vi "Live Capture Functional Stack.5.64bit.vi"() -> ()   [LabVIEW 2014]
uses:
  subvis/Stack Track.ctl
  subvis/Stack_State.ctl
  CameraControlTypeDef.ctl
  Desktop/camtiff/ctiff.llb/__CTIFFNewFileAndStyleUINT16.vi
  Desktop/camtiff/ctiff.llb/__CTIFFAddNewPageUINT16.vi
panel:
  in  "Slit Width / Lines 2":sgl=150.0
  out "Frame Index":i32
  in  "Temp":path=path "C:/temp.tmp"
  in  "Frames":i32=100
  in  "HardDisk Record":bool
  in  "Internal Line Interval":dbl
  in  "Slit Width / Lines":sgl=150.0
  in  "Camera Readout Mode":u16(ring)=12 items=["Full Frame"=1, "Slit Scanning"=12]
  in  "Readout Direction":sgl(ring)=1.0 items=["Forward"=1, "Backward"=2]
  in  "Trigger Mode":sgl(ring)=1.0 items=["Normal"=1, "Start "=6]
  in  "Trigger Source":sgl(ring)=2.0 items=["Internal"=1, "External"=2]
  out "State":T1=enum."Start Sequence"
  out "Image":u16[][](graph)
  out "Saving":bool
  in  "AutoIncrement":bool=TRUE
  in  "Path":path=path "C:/Users/spim/Desktop/Craig Cap/temp/a.tiff"
  in  "Frames":i32=100
  out "Frame Index":i32
  out "error out":errorcluster
  in  "stop":bool
  in  "Ram Record":bool
  out "Total Frames":i32
  out "Elapsed Time":u32
  out "Software FPS":dbl
  out "Camera FPS":dbl
  in  "H Offset":i32 min=0 max=0 step=4
  in  "H Width":i32 min=0 max=2048 step=4
  out "SMD":dbl
  out "SHO":i32
  in  "V Offset":i32 min=0 max=0 step=4
  in  "V Width":i32 min=0 max=2048 step=4
  in  "Binning":u16(ring) items=["1x1"=1, "2x2"=2, "4x4"=4]
  out "SHW":i32
  out "SVO":i32
  out "SVW":i32
  in  "Scan Mode":dbl min=0.0 max=2.0 step=1.0
  in  "Exposure":dbl min=0.0 max=10.000004210526315 step=1e-08
  out "EXP":dbl
  out "Camera Model":string
  out "Camera Version":string
  out "Camera Serial":string
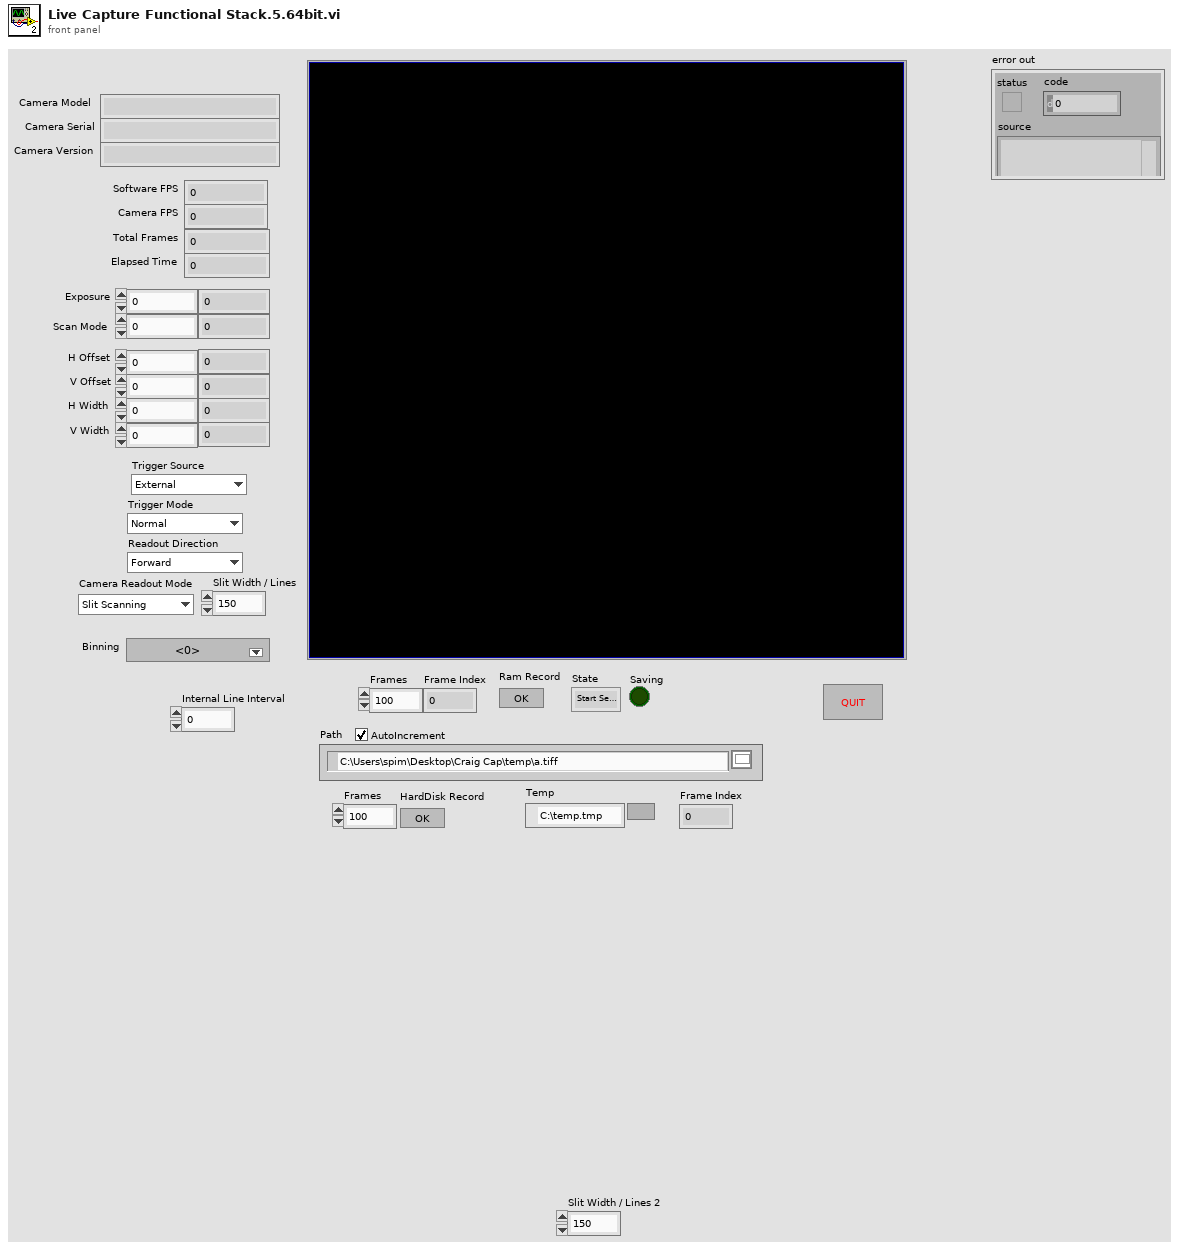
[diagram p1: front panel]
types:
  T1 = typedef "Stack Track.ctl" = enum16{"Idle", "Start Sequence", "Read Disk", "STOP", "Collecting", "End"}
  T2 = typedef "CameraControlTypeDef.ctl" = enum16{"Ram Record", "HardDisk Record", "Disengage Update", "Update", "Idle", "ROI", "Binning", "Scan Mode", "Trigger Mode", "Readout Mode", "Readout Direction"}
  T3 = typedef "Stack_State.ctl" = cluster{"State":T1, "Stack Number":i32, "Image":u16[][]}
  T4 = enum8{"Enabled", "Disabled", "Disabled and Grayed Out"}
  T5 = cluster{"Model":string, "Camera ID":string, "Firmware":string}
  T6 = cluster{"Value":i32, "Minimum":i32, "Maximum":i32, "Increment":i32}
  T7 = cluster{"height":u32, "width":u32, "datatype":u32}
  T8 = cluster{"H Offset":i32, "V Offset":i32, "H Width":i32, "V Width":i32}
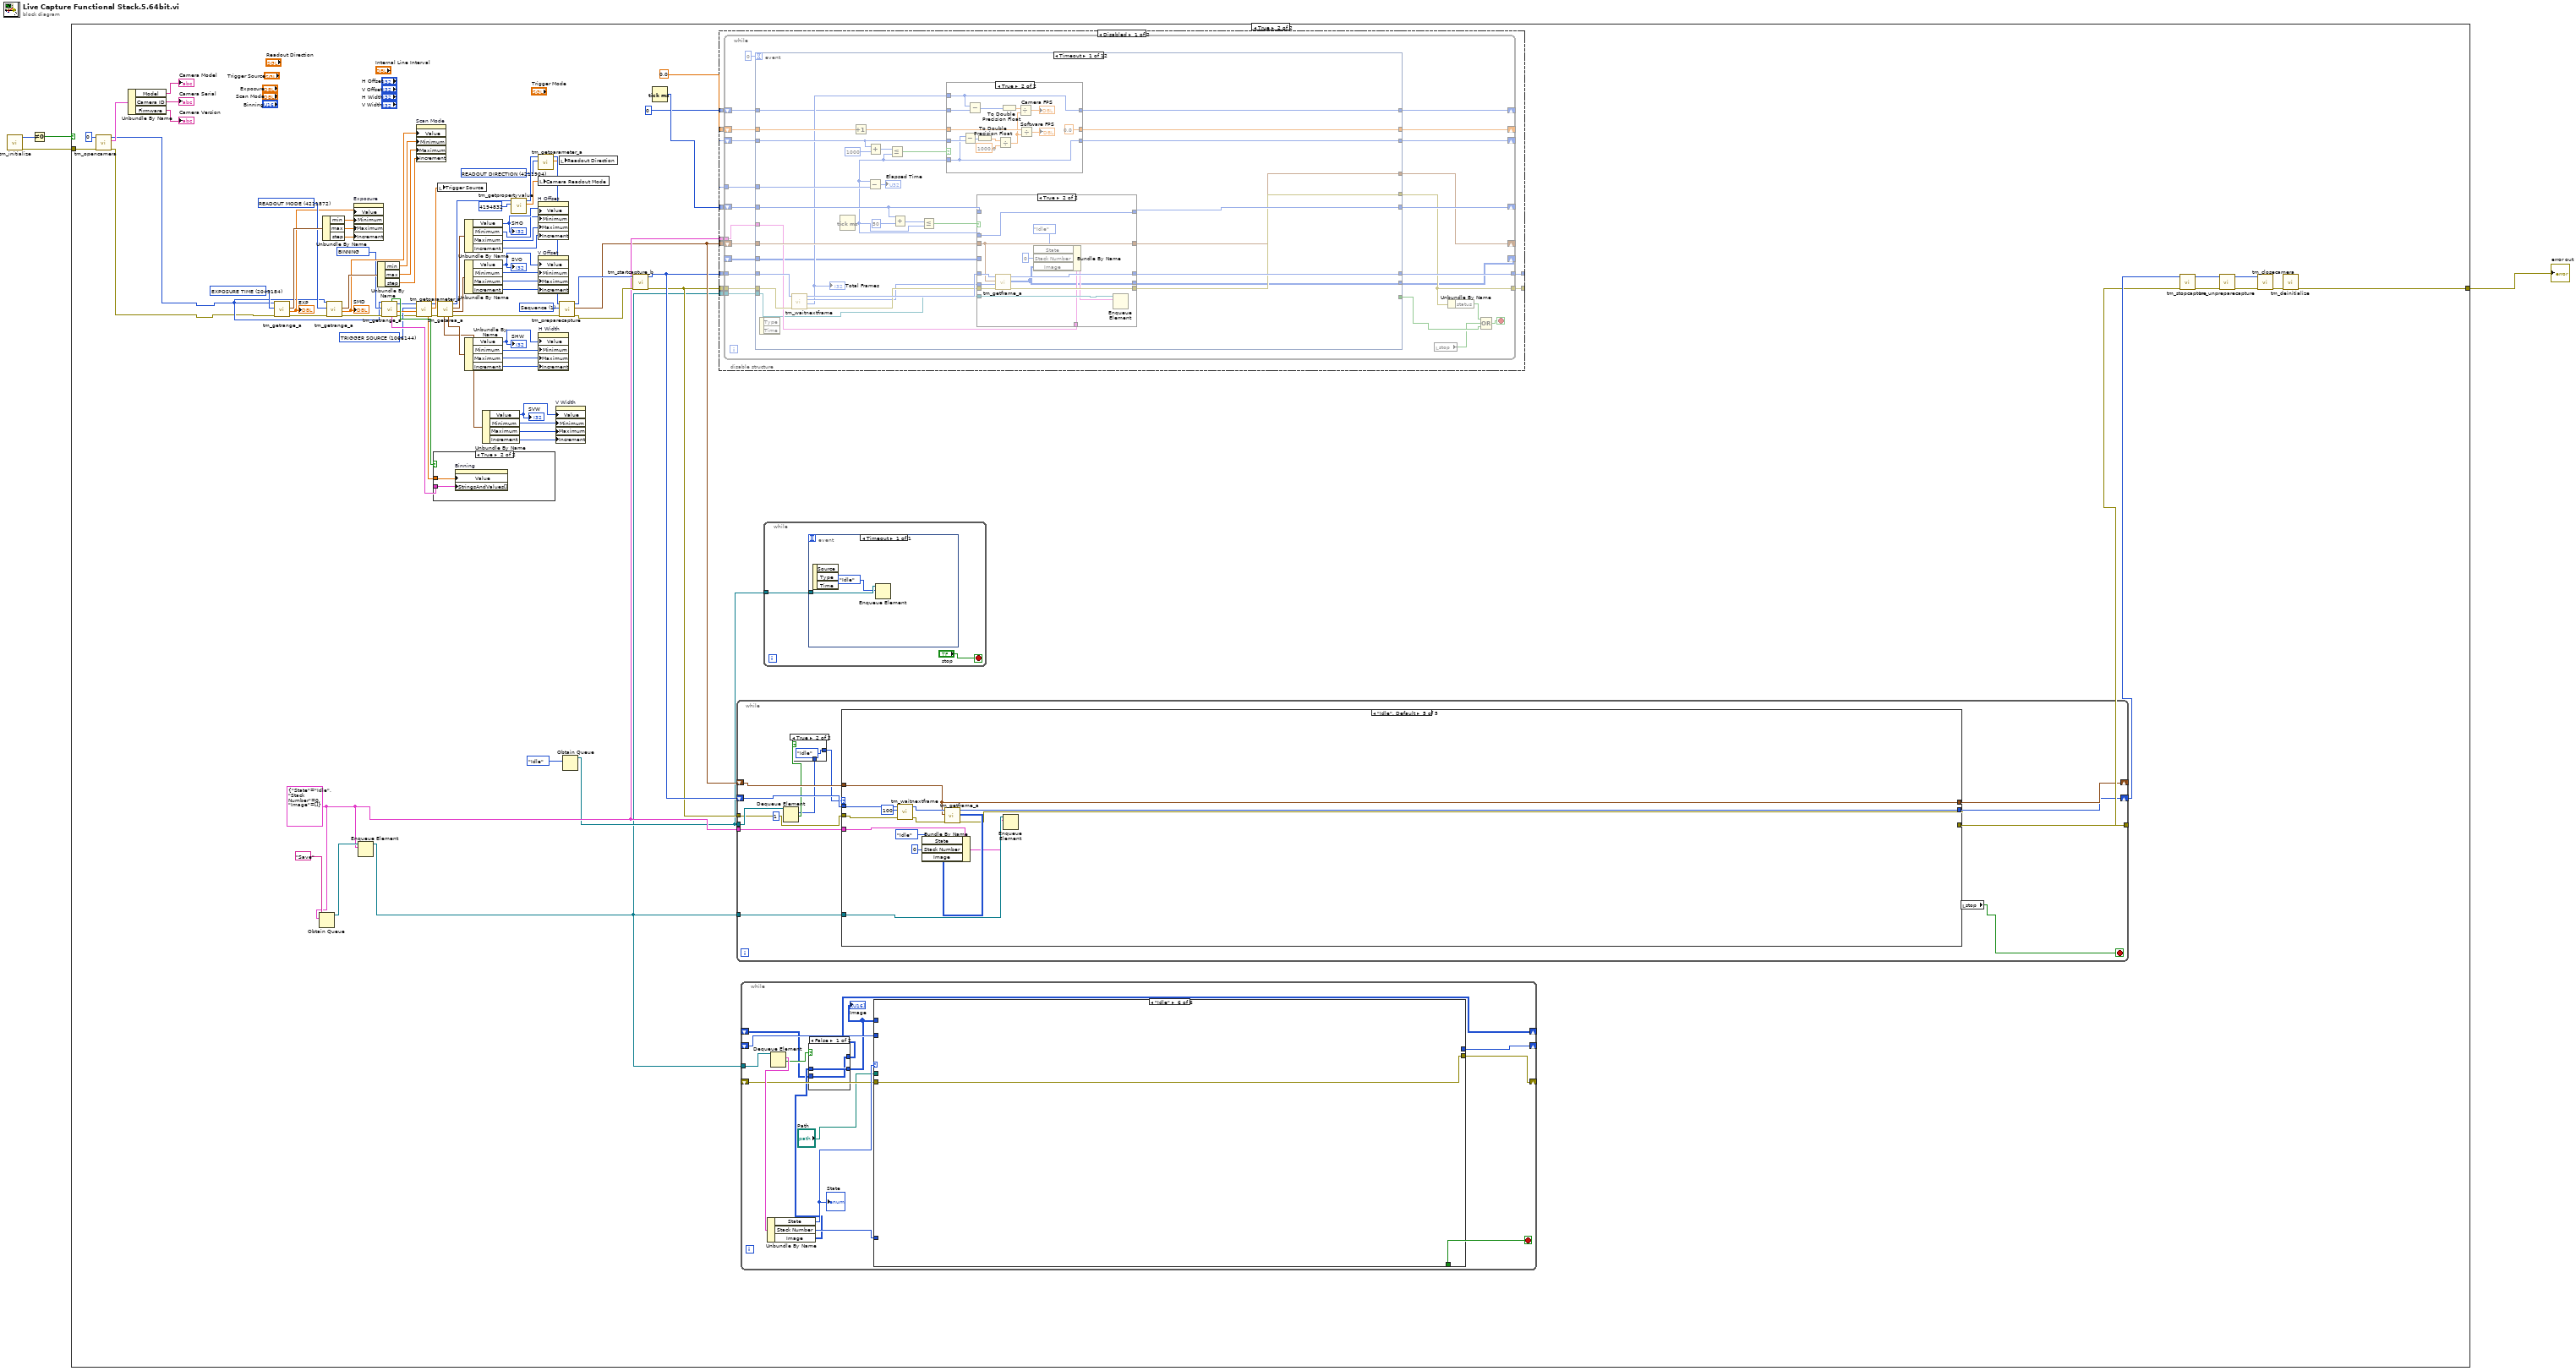
[diagram p0: block diagram]
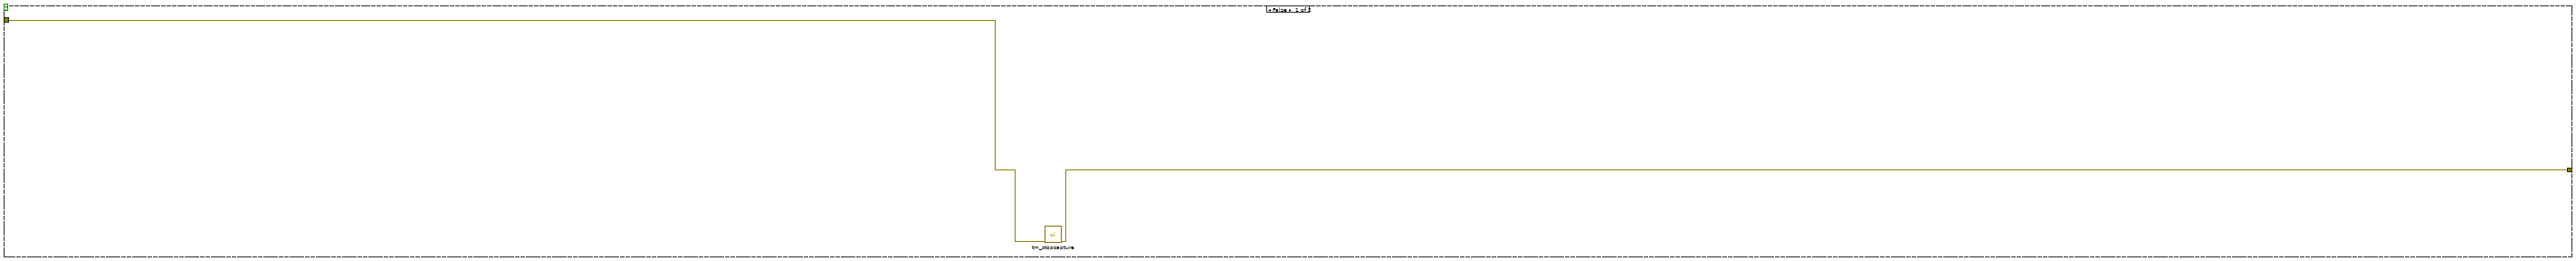
[diagram p2: hidden frame]
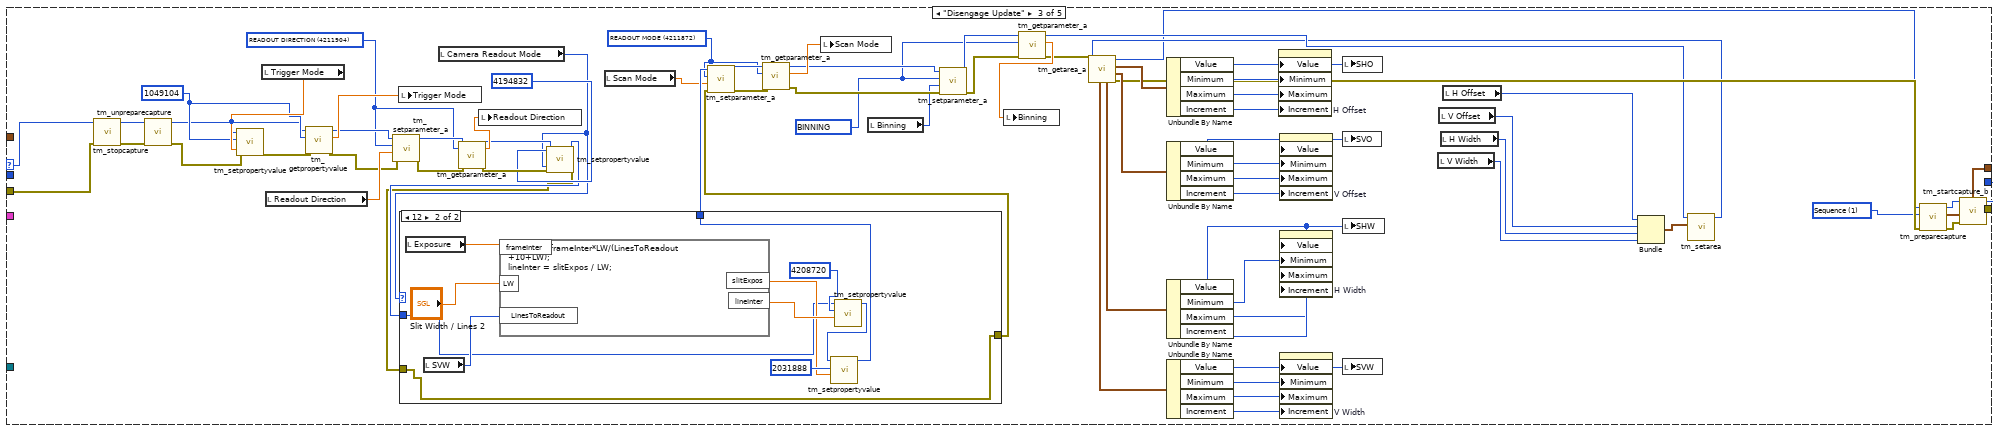
[diagram p6: hidden frame]
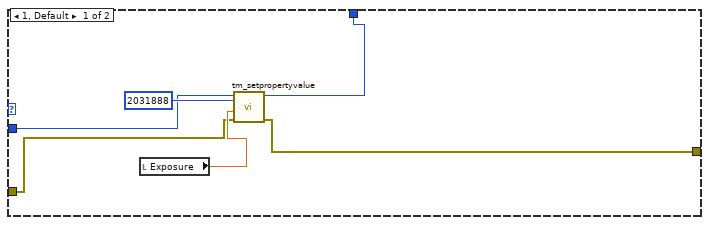
[diagram p7: hidden frame]
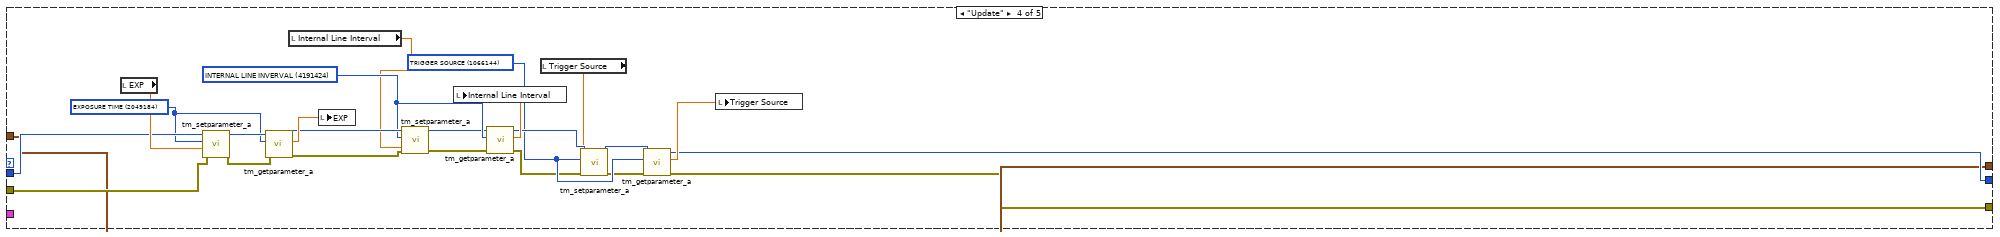
[diagram p8: hidden frame]
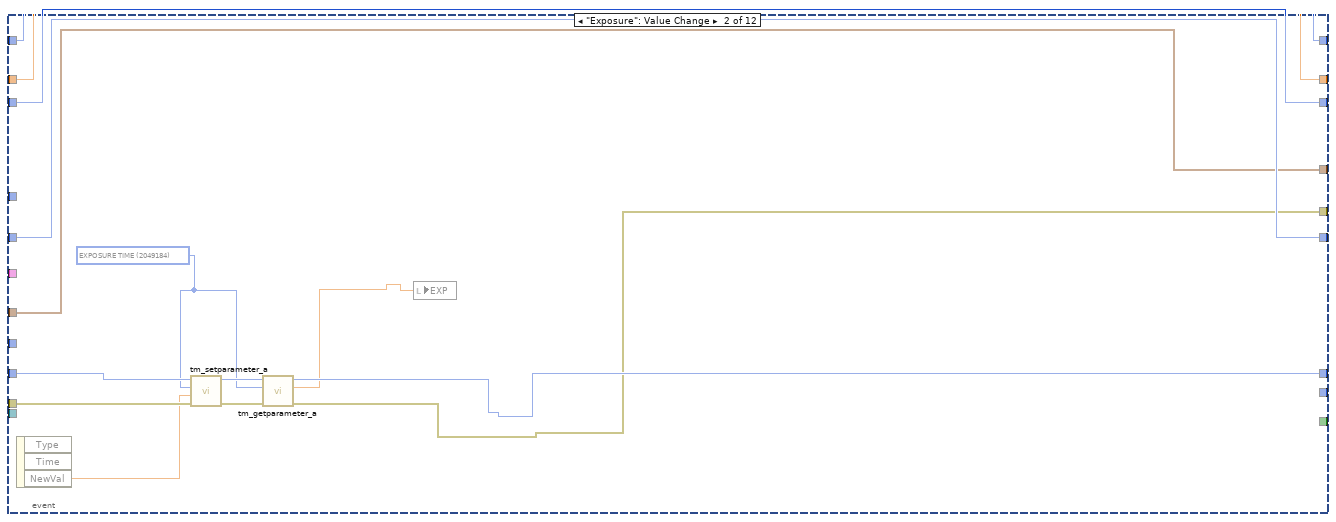
[diagram p11: hidden frame]
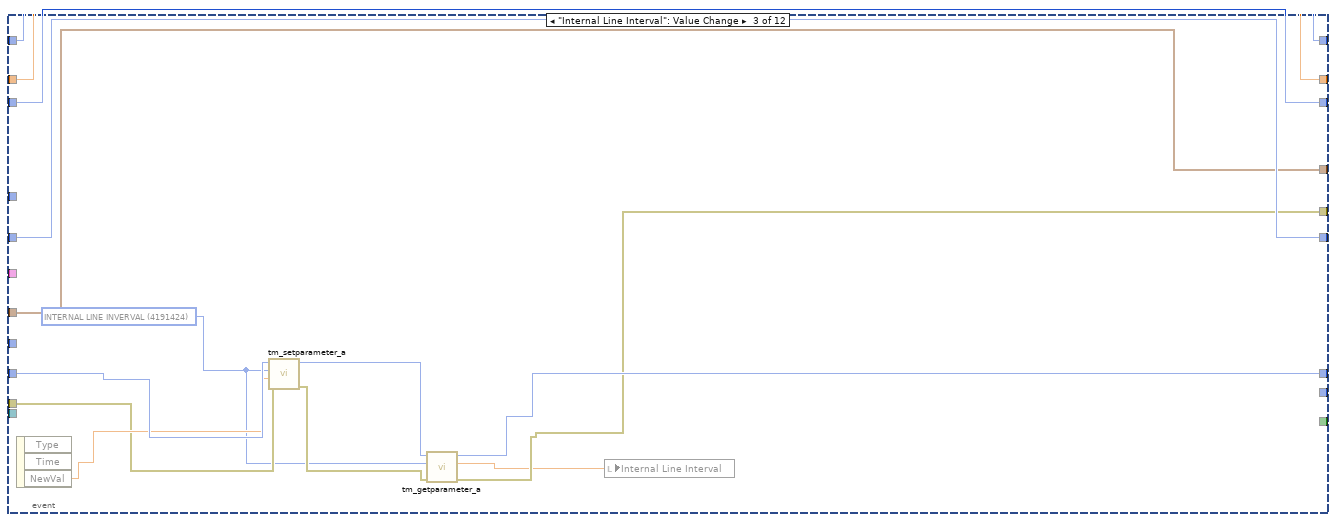
[diagram p12: hidden frame]
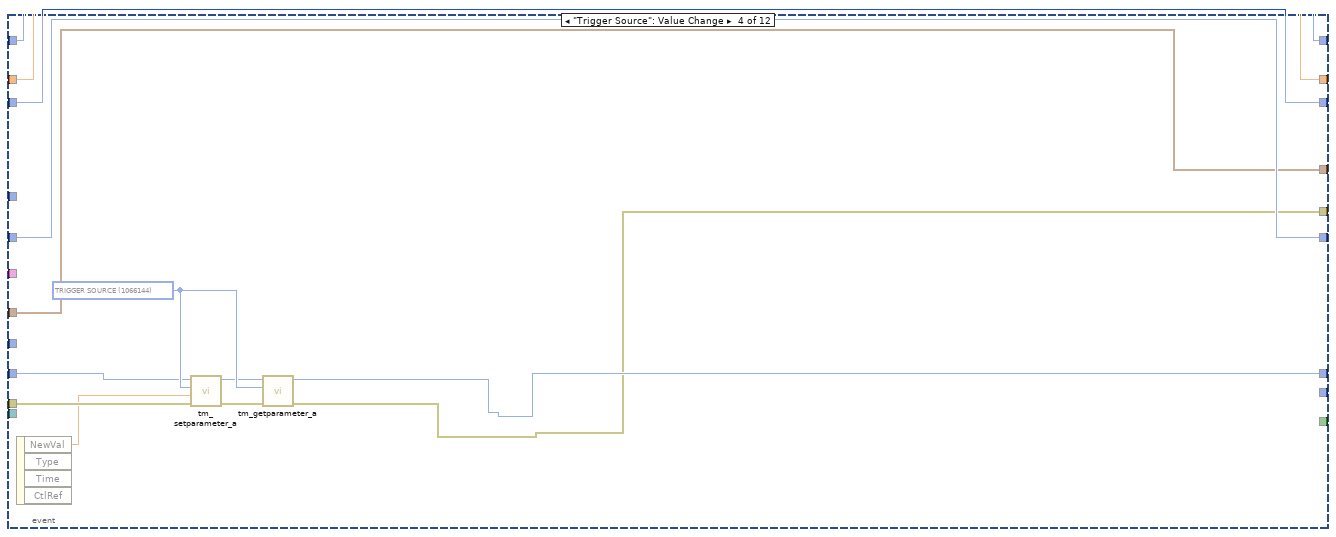
[diagram p13: hidden frame]
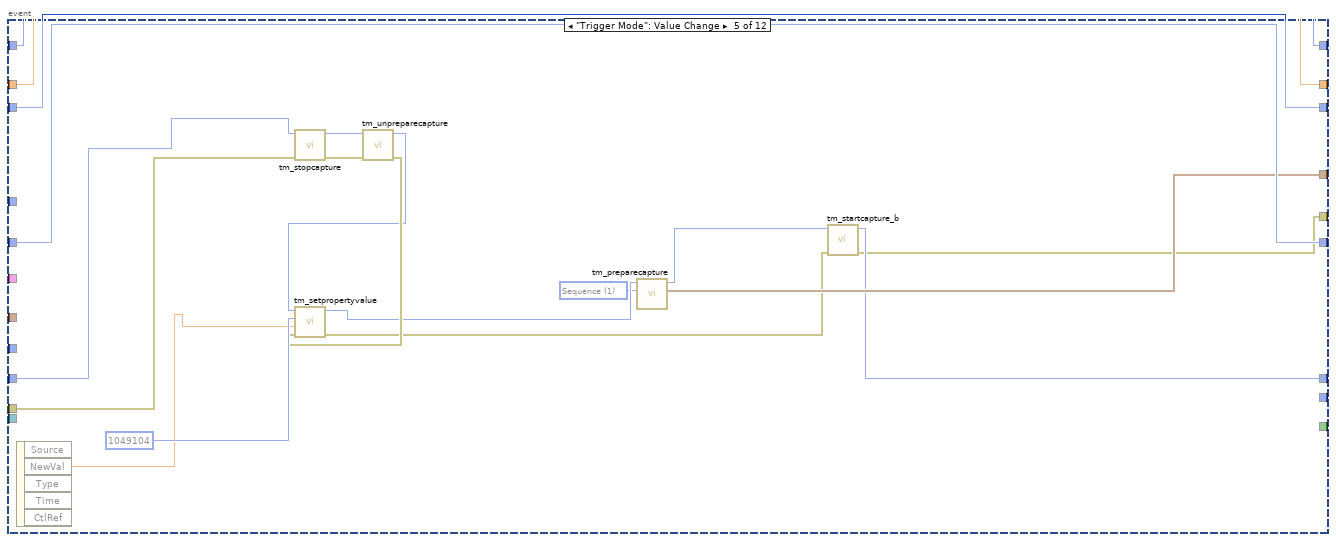
[diagram p14: hidden frame]
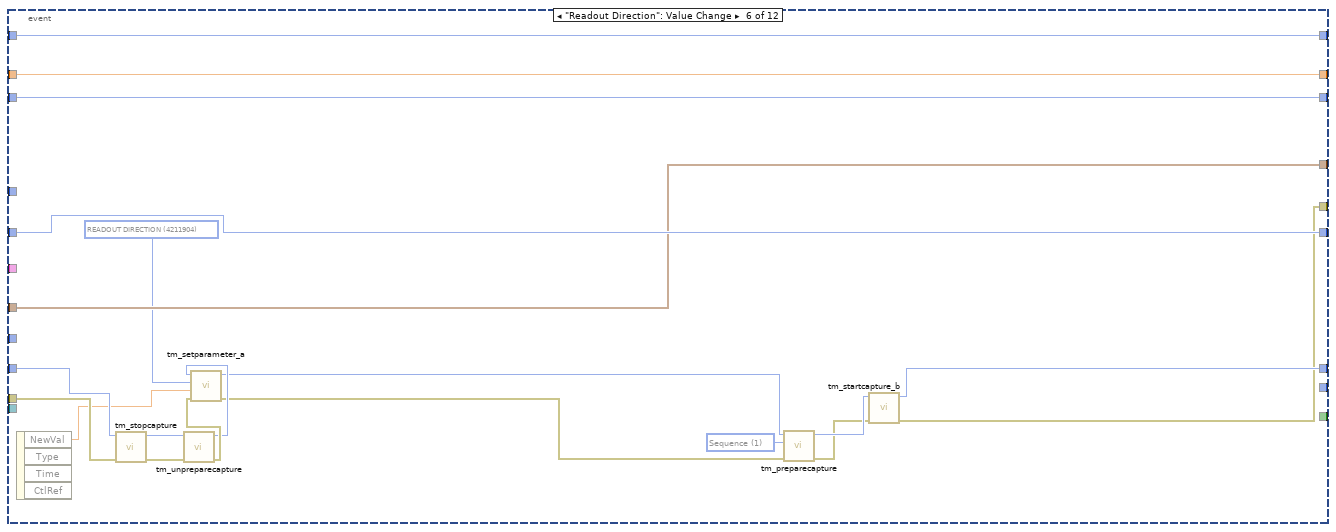
[diagram p15: hidden frame]
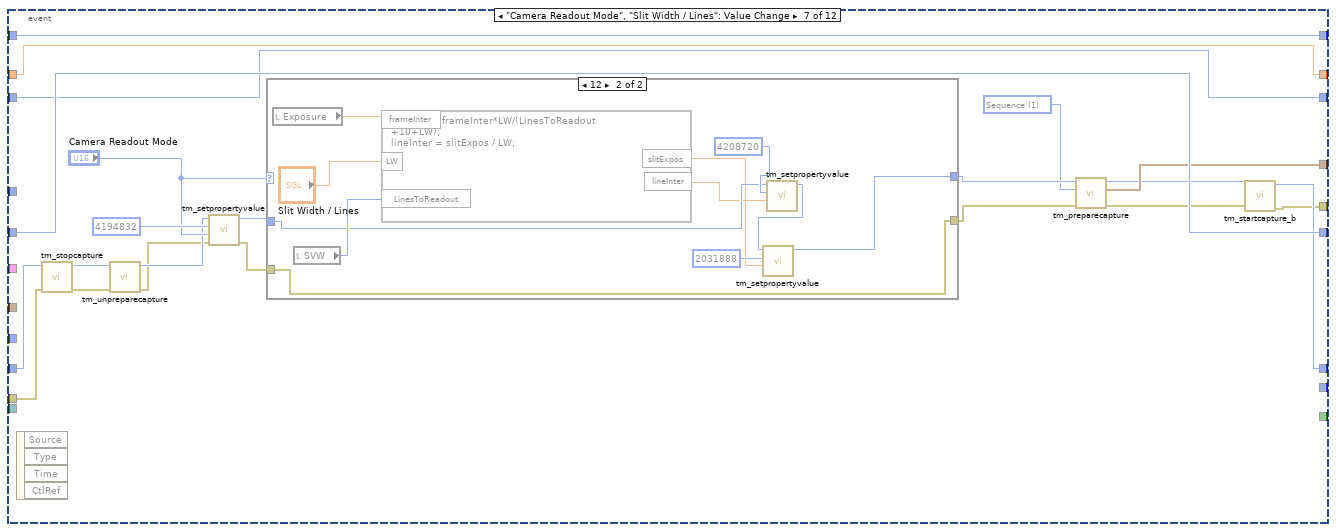
[diagram p16: hidden frame]
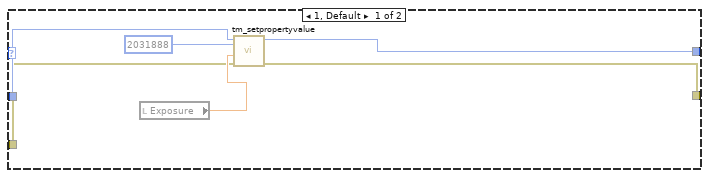
[diagram p17: hidden frame]
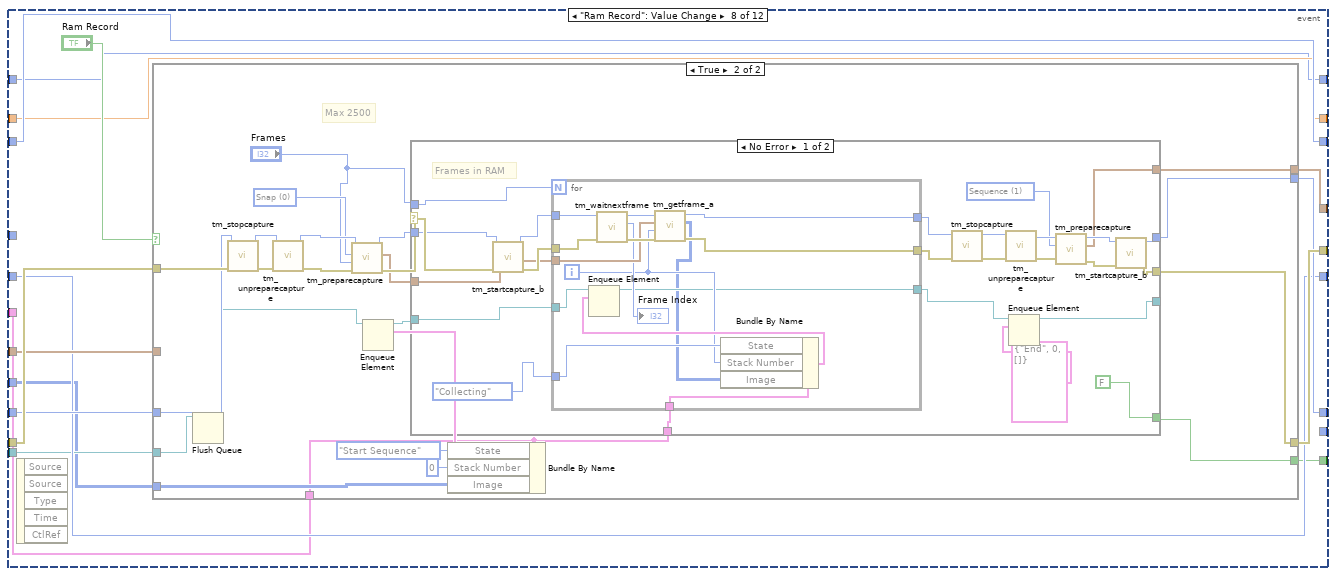
[diagram p18: hidden frame]
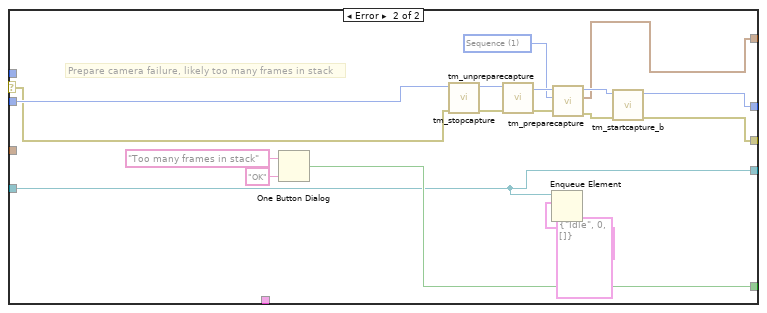
[diagram p20: hidden frame]
diagram:
  n1 = call <userlib>:"tm_initialize.vi"() -> ("error out"=w2:errorcluster, "Number Of Cameras"=w1:u32)  [unwired: 8 in, 2 out]
  n2 = Not Equal To 0?(x=w1) -> (x != 0?=w4:bool)
  n3 = case shown="True" w4 {
    tunnel: [w5 w86] -> w3
    tunnel: w2 -> [w6 w89]
    frame False {
      n4 = call <userlib>:"tm_stopcapture.vi"("error in (no error)"=w6) -> ("error out"=w5:errorcluster)  [unwired: 9 in, 1 out]
    }
    frame True {
      w22 = u32 4211904 items=["SENSOR MODE"=4212128, "CCD MODE"=4212384, "READOUT MODE"=4211872, "ACTIVE VIEW INDEX"=4343136, "BITS PER CHANNEL"=4342976, "IMAGE PIXEL TYPE"=4343296, "BINNING"=4215968, "EXPOSURE TIME"=2049184, "CONTRAST GAIN"=3163312, "CONTRAST OFFSET"=3163328, "LIGHT MODE"=2114720, "SENSITIVITY"=2114992, "PHOTON IMAGING MODE"=2115200, "HIGH DYNAMIC RANGE MODE"=3163360, "WHITE BALANCE"=3163568, "TEMPERATURE"=2115232, "TEMPERATURE TARGET"=2115264, "SENSOR COOLER FAN"=2115296, "LINEBUNDLE HEIGHT"=4212192, "MECHANICAL SHUTTER"=2115488, "BACK FOCUS POSITION"=8422304, "TRIGGER CONNECTOR"=1066432, "TRIGGER SOURCE"=1066144, "OUTPUT TRIGGER SOURCE"=1852576, "TRIGGER GLOBAL EXPOSURE"=2049680, "FIRST TRIGGER BEHAVIOR"=2049696, "CHANNEL SYNC"=1852352, "READOUT DIRECTION"=4211904, "PRE HSYNC COUNT"=1852704] ("Parameter")
      w32 = u32 1066144 items=["SENSOR MODE"=4212128, "CCD MODE"=4212384, "READOUT MODE"=4211872, "ACTIVE VIEW INDEX"=4343136, "BITS PER CHANNEL"=4342976, "IMAGE PIXEL TYPE"=4343296, "BINNING"=4215968, "EXPOSURE TIME"=2049184, "CONTRAST GAIN"=3163312, "CONTRAST OFFSET"=3163328, "LIGHT MODE"=2114720, "SENSITIVITY"=2114992, "PHOTON IMAGING MODE"=2115200, "HIGH DYNAMIC RANGE MODE"=3163360, "WHITE BALANCE"=3163568, "TEMPERATURE"=2115232, "TEMPERATURE TARGET"=2115264, "SENSOR COOLER FAN"=2115296, "LINEBUNDLE HEIGHT"=4212192, "MECHANICAL SHUTTER"=2115488, "BACK FOCUS POSITION"=8422304, "TRIGGER CONNECTOR"=1066432, "TRIGGER SOURCE"=1066144, "OUTPUT TRIGGER SOURCE"=1852576, "TRIGGER GLOBAL EXPOSURE"=2049680, "FIRST TRIGGER BEHAVIOR"=2049696, "CHANNEL SYNC"=1852352, "READOUT DIRECTION"=4211904, "PRE HSYNC COUNT"=1852704] ("Parameter")
      w15 = T3 {"State"=enum."Idle", "Stack Number"=0, "Image"=[]} ("input cluster")
      w37 = u32 2049184 items=["BINNING"=4215968, "BITS PER CHANNEL"=4342976, "ACTIVE VIEW INDEX"=4343136, "CCD MODE"=4212384, "SENSOR MODE"=4212128, "READOUT MODE"=4211872, "EXPOSURE TIME"=2049184, "CONTRAST GAIN"=3163312, "CONTRAST OFFSET"=3163328, "LIGHT MODE"=2114720, "SENSITIVITY"=2114992, "WHITE BALANCE"=3163568, "PHOTON IMAGING MODE"=2115200, "HIGH DYNAMIC RANGE MODE"=3163360, "TRIGGER SOURCE"=1066144, "TRIGGER ACTIVE"=1066160, "TRIGGER MODE"=1066400, "TRIGGER POLARITY"=1066416, "TRIGGER GLOBAL EXPOSURE"=2049680, "FIRST TRIGGER BEHAVIOR"=2049696, "TRIGGER TIMES"=1066448, "OUTPUT TRIGGER POLARITY"=1852592, "OUTPUT TRIGGER DELAY"=1852624, "OUTPUT TRIGGER PERIOD"=1852640, "TEMPERATURE"=2115232, "TEMPERATURE TARGET"=2115264, "SENSOR COOLER FAN"=2115296, "MECHANICAL SHUTTER"=2115488, "BACK FOCUS POSITION"=8422304, "FRAMEBUNDLE MODE"=4346784, "FRAMEBUNDLE NUMBER"=4346800, "LINEBUNDLE HEIGHT"=4212192, "TRIGGER CONNECTOR"=1066432, "IMAGE PIXEL TYPE"=4343296, "OUTPUT TRIGGER KIND"=1852656, "READOUT DIRECTION"=4211904, "CHANNEL SYNC"=1852352] ("Parameter")
      w38 = u32 4211872 items=["BINNING"=4215968, "BITS PER CHANNEL"=4342976, "ACTIVE VIEW INDEX"=4343136, "CCD MODE"=4212384, "SENSOR MODE"=4212128, "READOUT MODE"=4211872, "EXPOSURE TIME"=2049184, "CONTRAST GAIN"=3163312, "CONTRAST OFFSET"=3163328, "LIGHT MODE"=2114720, "SENSITIVITY"=2114992, "WHITE BALANCE"=3163568, "PHOTON IMAGING MODE"=2115200, "HIGH DYNAMIC RANGE MODE"=3163360, "TRIGGER SOURCE"=1066144, "TRIGGER ACTIVE"=1066160, "TRIGGER MODE"=1066400, "TRIGGER POLARITY"=1066416, "TRIGGER GLOBAL EXPOSURE"=2049680, "FIRST TRIGGER BEHAVIOR"=2049696, "TRIGGER TIMES"=1066448, "OUTPUT TRIGGER POLARITY"=1852592, "OUTPUT TRIGGER DELAY"=1852624, "OUTPUT TRIGGER PERIOD"=1852640, "TEMPERATURE"=2115232, "TEMPERATURE TARGET"=2115264, "SENSOR COOLER FAN"=2115296, "MECHANICAL SHUTTER"=2115488, "BACK FOCUS POSITION"=8422304, "FRAMEBUNDLE MODE"=4346784, "FRAMEBUNDLE NUMBER"=4346800, "LINEBUNDLE HEIGHT"=4212192, "TRIGGER CONNECTOR"=1066432, "IMAGE PIXEL TYPE"=4343296, "OUTPUT TRIGGER KIND"=1852656, "READOUT DIRECTION"=4211904, "CHANNEL SYNC"=1852352] ("Parameter")
      w39 = u32 4215968 items=["BINNING"=4215968, "BITS PER CHANNEL"=4342976, "ACTIVE VIEW INDEX"=4343136, "CCD MODE"=4212384, "SENSOR MODE"=4212128, "READOUT MODE"=4211872, "EXPOSURE TIME"=2049184, "CONTRAST GAIN"=3163312, "CONTRAST OFFSET"=3163328, "LIGHT MODE"=2114720, "SENSITIVITY"=2114992, "WHITE BALANCE"=3163568, "PHOTON IMAGING MODE"=2115200, "HIGH DYNAMIC RANGE MODE"=3163360, "TRIGGER SOURCE"=1066144, "TRIGGER ACTIVE"=1066160, "TRIGGER MODE"=1066400, "TRIGGER POLARITY"=1066416, "TRIGGER GLOBAL EXPOSURE"=2049680, "FIRST TRIGGER BEHAVIOR"=2049696, "TRIGGER TIMES"=1066448, "OUTPUT TRIGGER POLARITY"=1852592, "OUTPUT TRIGGER DELAY"=1852624, "OUTPUT TRIGGER PERIOD"=1852640, "TEMPERATURE"=2115232, "TEMPERATURE TARGET"=2115264, "SENSOR COOLER FAN"=2115296, "MECHANICAL SHUTTER"=2115488, "BACK FOCUS POSITION"=8422304, "FRAMEBUNDLE MODE"=4346784, "FRAMEBUNDLE NUMBER"=4346800, "LINEBUNDLE HEIGHT"=4212192, "TRIGGER CONNECTOR"=1066432, "IMAGE PIXEL TYPE"=4343296, "OUTPUT TRIGGER KIND"=1852656, "READOUT DIRECTION"=4211904, "CHANNEL SYNC"=1852352] ("Parameter")
      w84 = 1 items=["Snap", "Sequence"] ("Capture mode")
      n5 = call <userlib>:"tm_opencamera.vi"("error in (no error)"=w89, "Camera Index"=u32 0) -> ("error out"=w16:errorcluster, "Camera Details"=w51:T5, "Handle out"=w17:u32)  [unwired: 7 in]
      n6 = Unbundle By Name(w51) -> ("Model"=→"Camera Model":string, "Camera ID"=→"Camera Serial":string, "Firmware"=→"Camera Version":string)
      n7 = call <userlib>:"tm_getrange_a.vi"("error in (no error)"=w16, "Parameter"=w37, "Handle in"=w17) -> ("error out"=w46:errorcluster, "default"=w35:dbl, "Range"=w47:cluster{"min":dbl, "max":dbl, "step":dbl})  [unwired: 2 in, 4 out]
      "EXP" <- w35
      n8 = Obtain Queue(name (unnamed)="Save", element data type=w15) -> (queue out=w19:refnum<queue>)  [unwired: 3 in, 2 out]
      n9 = Unbundle By Name(w47) -> ("min"=w82:dbl, "max"=w81:dbl, "step"=w80:dbl)
      n10 = call <userlib>:"tm_getrange_a.vi"("error in (no error)"=w46, "Parameter"=w38, "Handle in"=w17) -> ("error out"=w43:errorcluster, "default"=w44:dbl, "Range"=w45:cluster{"min":dbl, "max":dbl, "step":dbl})  [unwired: 2 in, 4 out]
      "SMD" <- w44
      n11 = property on="Exposure" class="DigNum (strict)"("Value"=w35, "Minimum"=w82, "Maximum"=w81, "Increment"=w80) -> ()  [unwired: 2 in, 2 out]
      n12 = Enqueue Element(queue=w19, element=w15) -> (queue out=w9:refnum<queue>)  [unwired: 2 in, 2 out]
      n13 = Unbundle By Name(w45) -> ("min"=w79:dbl, "max"=w78:dbl, "step"=w77:dbl)
      n14 = call <userlib>:"tm_getrange_a.vi"("error in (no error)"=w43, "Parameter"=w39, "Handle in"=w17) -> ("error out"=w29:errorcluster, "default"=w41:dbl, "Handle out"=w31:u32, "Value Names"=w40:cluster{"Name":string, "Value":dbl}[], "Writable"=w42:bool)  [unwired: 2 in, 2 out]
      n15 = property on="Scan Mode" class="DigNum (strict)"("Value"=w44, "Minimum"=w79, "Maximum"=w78, "Increment"=w77) -> ()  [unwired: 2 in, 2 out]
      n16 = call <userlib>:"tm_getparameter_a.vi"("error in (no error)"=w29, "Parameter"=w32, "Handle in"=w31) -> ("error out"=w28:errorcluster, "Value out"=w33:dbl, "Handle out"=w30:u32)  [unwired: 6 in]
      n17 = case shown="True" w42 {
        tunnel: w40 -> [_ w837]
        tunnel: w41 -> [_ w836]
        frame False {
        }
        frame True {
          n18 = property on="Binning" class="Ring (strict)"("Value"=w836, "StringsAndValues[]"=w837) -> ()  [unwired: 2 in, 2 out]
        }
      }
      n19 = local write "Trigger Source"(w33) -> ()
      n20 = call <userlib>:"tm_getarea_a.vi"("error in (no error)"=w28, "Handle in"=w30) -> ("error out"=w34:errorcluster, "V Offset"=w76:T6, "H Offset"=w57:T6, "Handle out"=w25:u32, "H Width"=w75:T6, "V Width"=w74:T6)  [unwired: 4 in]
      n21 = Unbundle By Name(w57) -> ("Value"=w56:i32, "Minimum"=w55:i32, "Maximum"=w54:i32, "Increment"=w53:i32)
      "SHO" <- w56
      n22 = Unbundle By Name(w76) -> ("Value"=w64:i32, "Minimum"=w73:i32, "Maximum"=w72:i32, "Increment"=w71:i32)
      "SVO" <- w64
      n23 = Unbundle By Name(w75) -> ("Value"=w63:i32, "Minimum"=w70:i32, "Maximum"=w69:i32, "Increment"=w68:i32)
      "SHW" <- w63
      n24 = Unbundle By Name(w74) -> ("Value"=w62:i32, "Minimum"=w67:i32, "Maximum"=w66:i32, "Increment"=w65:i32)
      "SVW" <- w62
      n25 = call <userlib>:"tm_getpropertyvalue.vi"("Property ID"=u32 4194832, "Handle in"=w25) -> ("Value in"=w26:sgl, "Handle out"=w24:u32)  [unwired: 7 in, 1 out]
      n26 = call <userlib>:"tm_getparameter_a.vi"("Parameter"=w22, "Handle in"=w24) -> ("Value out"=w21:dbl, "Handle out"=w23:u32)  [unwired: 7 in, 1 out]
      n27 = local write "Camera Readout Mode"(w26) -> ()
      n28 = property on="H Offset" class="DigNum (strict)"("Value"=w56, "Minimum"=w55, "Maximum"=w54, "Increment"=w53) -> ()  [unwired: 2 in, 2 out]
      n29 = property on="V Offset" class="DigNum (strict)"("Value"=w64, "Minimum"=w73, "Maximum"=w72, "Increment"=w71) -> ()  [unwired: 2 in, 2 out]
      n30 = property on="H Width" class="DigNum (strict)"("Value"=w63, "Minimum"=w70, "Maximum"=w69, "Increment"=w68) -> ()  [unwired: 2 in, 2 out]
      n31 = property on="V Width" class="DigNum (strict)"("Value"=w62, "Minimum"=w67, "Maximum"=w66, "Increment"=w65) -> ()  [unwired: 2 in, 2 out]
      n32 = local write "Readout Direction"(w21) -> ()
      n33 = call <userlib>:"tm_preparecapture.vi"("error in (no error)"=w34, "Capture mode"=w84, "Handle in"=w23) -> ("error out"=w18:errorcluster, "Buffer Info"=w14:T7, "Handle out"=w20:u32)  [unwired: 5 in, 1 out]
      n34 = Obtain Queue(element data type=CameraControlTypeDef."Idle" ("Enum")) -> (queue out=w10:refnum<queue>)  [unwired: 4 in, 2 out]
      n35 = call <userlib>:"tm_startcapture_b.vi"("error in (no error)"=w18, "Handle in"=w20) -> ("error out"=w12:errorcluster, "Handle out"=w13:u32)  [unwired: 8 in]
      n36 = Tick Count (ms)() -> (millisecond timer value=w83:u32)
      n37 = disable-structure shown="Disabled" {
        disable-tunnel: 0.0 -> [w253 _]
        disable-tunnel: w83 -> [w252 _]
        disable-tunnel: 0 -> [w251 _]
        disable-tunnel: [w250 _] -> _
        disable-tunnel: [w249 _] -> _
        disable-tunnel: w15 -> [w248 _]
        disable-tunnel: w14 -> [w247 _]
        disable-tunnel: w13 -> [w246 _]
        disable-tunnel: w12 -> [w245 _]
        disable-tunnel: w9 -> [w244 _]
        frame Disabled {
          n38 = while {
            tunnel: w245 -> [w267]
            tunnel: [w265] -> w249
            tunnel: [w264] -> w250
            shift-right: [w274] -> _
            shift-left: w252 -> [w272]
            shift-right: [w275] -> _
            shift-left: w253 -> [w273]
            shift-right: [w266] -> _
            shift-left: w252 -> [w270]
            tunnel: w246 -> [w268]
            tunnel: w252 -> [w271]
            shift-right: [w263] -> _
            shift-left: w247 -> [w269]
            shift-right: [w261] -> _
            shift-left: w251 -> [w262]
            tunnel: w244 -> [w260]
            shift-right: [w258] -> _
            shift-left: _ -> [w257]
            tunnel: w248 -> [w256]
            stop <- w276 stop-if-true
            n39 = event shown="[0] Timeout" {
              selector: _ -> [_ _ _ _ _ _ _ _ _ _ _ _]
              dyn-events: _ -> [_ _ _ _ _ _ _ _ _ _ _ _]
              timeout: 0 -> [_ _ _ _ _ _ _ _ _ _ _ _]
              tunnel: [w287 w356 w370 w383 w402 w422 w444 w472 w569 w663 w699 w744] -> w275
              tunnel: [w286 w357 w371 w384 w403 w423 w445 w473 w570 w664 w700 w745] -> w274
              tunnel: w273 -> [w298 w356 w370 w383 w402 w422 w444 w472 w569 w663 w699 w744]
              tunnel: w272 -> [w289 w357 w371 w384 w403 w423 w445 w473 w570 w664 w700 w745]
              tunnel: w271 -> [w294 _ _ _ _ _ _ _ _ _ _ _]
              tunnel: w270 -> [w299 w358 w372 w385 w404 w424 w446 w468 w565 w665 w707 w752]
              tunnel: w269 -> [w293 w355 w369 w382 _ w421 _ w469 w566 _ _ _]
              tunnel: w268 -> [w301 w351 w364 w378 w397 w415 w437 w476 w573 w660 w676 w714]
              tunnel: w267 -> [w300 w353 w360 w379 w396 w418 w436 w477 w574 w659 w675 w713]
              tunnel: [w297 w358 w372 w385 w404 w424 w446 w468 w565 w665 w707 w752] -> w266
              tunnel: [w296 w348 w367 w375 w388 w408 w427 w474 w571 w654 w702 w747] -> w265
              tunnel: [w295 w347 w366 w374 w387 w407 w425 w475 w572 w655 w703 w748] -> w264
              tunnel: [w292 w355 w369 w382 w391 w421 w432 w470 w567 w653 w701 w746] -> w263
              tunnel: w262 -> [w284 w354 w368 w381 w401 w420 w443 w471 w568 w652 w672 w708]
              tunnel: [w283 w354 w368 w381 w401 w420 w443 w471 w568 w652 w672 w708] -> w261
              tunnel: w260 -> [w278 _ _ _ _ _ _ w467 w564 _ _ _]
              tunnel: [_ _ _ _ _ _ _ w466 w563 _ _ _] -> w259
              tunnel: w256 -> [w281 _ _ _ _ _ _ w464 _ _ _ _]
              tunnel: [w280 _ _ _ _ _ _ _ _ _ _ _] -> w258
              tunnel: w257 -> [w279 _ _ _ _ _ _ w465 _ _ _ _]
              event Timeout {
                n40 = event-data() -> ()  [unwired: 1 in, 2 out]
                n41 = call <userlib>:"tm_waitnextframe.vi"("error in (no error)"=w300, "Handle in"=w301) -> ("error out"=w304:errorcluster, "Frame Count"=w285:i32, "Frame Index"=w303:i32, "Handle out"=w305:u32)  [unwired: 6 in]
                "Total Frames" <- w285
                n42 = Tick Count (ms)() -> (millisecond timer value=w291:u32)
                n43 = Increment(x=w298) -> (x+1=w288:dbl)
                n44 = Subtract(x=w291, y=w294) -> (x-y=→"Elapsed Time":u32)
                n45 = Add(x=w289, y=u32 1000) -> (x+y=w309:u32)
                n46 = Less Or Equal?(x=w309, y=w291) -> (x <= y?=w290:bool)
                n47 = Add(x=w299, y=u32 50) -> (x+y=w307:u32)
                n48 = Less Or Equal?(x=w307, y=w291) -> (x <= y?=w282:bool)
                n49 = case shown="True" w290 {
                  tunnel: w289 -> [w312 w321]
                  tunnel: [w312 w318] -> w286
                  tunnel: w288 -> [w311 w324]
                  tunnel: w291 -> [_ w318]
                  tunnel: [w311 0.0] -> w287
                  tunnel: w285 -> [_ w313]
                  tunnel: w284 -> [w310 w316]
                  tunnel: [w310 w313] -> w283
                  frame False {
                  }
                  frame True {
                    n50 = Subtract(x=w318, y=w321) -> (x-y=w320:u32)
                    n51 = Subtract(x=w313, y=w316) -> (x-y=w314:i32)
                    n52 = To Double Precision Float(number=w320) -> (double precision float=w326:dbl)
                    n53 = Divide(x=w326, y=1000.0) -> (x/y=w317:dbl)
                    n54 = To Double Precision Float(number=w314) -> (double precision float=w315:dbl)
                    n55 = Divide(x=w315, y=w317) -> (x/y=→"Camera FPS":dbl)
                    n56 = Divide(x=w324, y=w317) -> (x/y=→"Software FPS":dbl)
                  }
                }
                n57 = case shown="True" w282 {
                  tunnel: w299 -> [w331 _]
                  tunnel: w291 -> [_ w344]
                  tunnel: [w331 w344] -> w297
                  tunnel: w305 -> [w330 w343]
                  tunnel: w293 -> [w328 w338]
                  tunnel: w304 -> [w329 w342]
                  tunnel: [w330 w341] -> w296
                  tunnel: [w329 w340] -> w295
                  tunnel: w303 -> [_ w339]
                  tunnel: [w328 w338] -> w292
                  tunnel: w278 -> [_ w337]
                  tunnel: w281 -> [_ w333]
                  tunnel: [w327 w332] -> w280
                  tunnel: w279 -> [w327 _]
                  frame False {
                  }
                  frame True {
                    n58 = call <userlib>:"tm_getframe_a.vi"("error in (no error)"=w342, "Frame Index"=w339, "Buffer Info"=w338, "Handle in"=w343) -> ("error out"=w340:errorcluster, "Data 16"=w332:u16[][], "Handle out"=w341:u32)  [unwired: 3 in, 2 out]
                    n59 = Bundle By Name(cluster=w333, "State"=Stack_Track."Idle", "Stack Number"=0, "Image"=w332) -> (w334:T3)
                    n60 = Enqueue Element(queue=w337, element=w334) -> ()  [unwired: 2 in, 3 out]
                  }
                }
              }
              event "Exposure": Value Change {
                w346 = u32 2049184 items=["SENSOR MODE"=4212128, "CCD MODE"=4212384, "READOUT MODE"=4211872, "ACTIVE VIEW INDEX"=4343136, "BITS PER CHANNEL"=4342976, "IMAGE PIXEL TYPE"=4343296, "BINNING"=4215968, "EXPOSURE TIME"=2049184, "CONTRAST GAIN"=3163312, "CONTRAST OFFSET"=3163328, "LIGHT MODE"=2114720, "SENSITIVITY"=2114992, "PHOTON IMAGING MODE"=2115200, "HIGH DYNAMIC RANGE MODE"=3163360, "WHITE BALANCE"=3163568, "TEMPERATURE"=2115232, "TEMPERATURE TARGET"=2115264, "SENSOR COOLER FAN"=2115296, "LINEBUNDLE HEIGHT"=4212192, "MECHANICAL SHUTTER"=2115488, "BACK FOCUS POSITION"=8422304, "TRIGGER CONNECTOR"=1066432, "TRIGGER SOURCE"=1066144, "OUTPUT TRIGGER SOURCE"=1852576, "TRIGGER GLOBAL EXPOSURE"=2049680, "FIRST TRIGGER BEHAVIOR"=2049696, "CHANNEL SYNC"=1852352, "READOUT DIRECTION"=4211904, "PRE HSYNC COUNT"=1852704] ("Parameter")
                n61 = event-data() -> ("NewVal"=w352:dbl)  [unwired: 1 in, 2 out]
                n62 = call <userlib>:"tm_setparameter_a.vi"("error in (no error)"=w353, "Value in"=w352, "Parameter"=w346, "Handle in"=w351) -> ("error out"=w350:errorcluster, "Handle out"=w349:u32)  [unwired: 6 in]
                n63 = call <userlib>:"tm_getparameter_a.vi"("error in (no error)"=w350, "Parameter"=w346, "Handle in"=w349) -> ("error out"=w347:errorcluster, "Value out"=w345:dbl, "Handle out"=w348:u32)  [unwired: 6 in]
                n64 = local write "EXP"(w345) -> ()
              }
              event "Internal Line Interval": Value Change {
                w359 = u32 4191424 items=["SENSOR MODE"=4212128, "CCD MODE"=4212384, "READOUT MODE"=4211872, "ACTIVE VIEW INDEX"=4343136, "BITS PER CHANNEL"=4342976, "IMAGE PIXEL TYPE"=4343296, "BINNING"=4215968, "EXPOSURE TIME"=2049184, "CONTRAST GAIN"=3163312, "CONTRAST OFFSET"=3163328, "LIGHT MODE"=2114720, "SENSITIVITY"=2114992, "PHOTON IMAGING MODE"=2115200, "HIGH DYNAMIC RANGE MODE"=3163360, "WHITE BALANCE"=3163568, "TEMPERATURE"=2115232, "TEMPERATURE TARGET"=2115264, "SENSOR COOLER FAN"=2115296, "LINEBUNDLE HEIGHT"=4212192, "MECHANICAL SHUTTER"=2115488, "BACK FOCUS POSITION"=8422304, "TRIGGER CONNECTOR"=1066432, "TRIGGER SOURCE"=1066144, "OUTPUT TRIGGER SOURCE"=1852576, "TRIGGER GLOBAL EXPOSURE"=2049680, "FIRST TRIGGER BEHAVIOR"=2049696, "CHANNEL SYNC"=1852352, "READOUT DIRECTION"=4211904, "PRE HSYNC COUNT"=1852704, "INTERNAL LINE SPEED"=4191408, "INTERNAL LINE INVERVAL"=4191424] ("Parameter")
                n65 = event-data() -> ("NewVal"=w363:dbl)  [unwired: 1 in, 2 out]
                n66 = call <userlib>:"tm_setparameter_a.vi"("error in (no error)"=w360, "Value in"=w363, "Parameter"=w359, "Handle in"=w364) -> ("error out"=w361:errorcluster, "Handle out"=w362:u32)  [unwired: 6 in]
                n67 = call <userlib>:"tm_getparameter_a.vi"("error in (no error)"=w361, "Parameter"=w359, "Handle in"=w362) -> ("error out"=w366:errorcluster, "Value out"=w365:dbl, "Handle out"=w367:u32)  [unwired: 6 in]
                n68 = local write "Internal Line Interval"(w365) -> ()
              }
              event "Trigger Source": Value Change {
                w380 = u32 1066144 items=["SENSOR MODE"=4212128, "CCD MODE"=4212384, "READOUT MODE"=4211872, "ACTIVE VIEW INDEX"=4343136, "BITS PER CHANNEL"=4342976, "IMAGE PIXEL TYPE"=4343296, "BINNING"=4215968, "EXPOSURE TIME"=2049184, "CONTRAST GAIN"=3163312, "CONTRAST OFFSET"=3163328, "LIGHT MODE"=2114720, "SENSITIVITY"=2114992, "PHOTON IMAGING MODE"=2115200, "HIGH DYNAMIC RANGE MODE"=3163360, "WHITE BALANCE"=3163568, "TEMPERATURE"=2115232, "TEMPERATURE TARGET"=2115264, "SENSOR COOLER FAN"=2115296, "LINEBUNDLE HEIGHT"=4212192, "MECHANICAL SHUTTER"=2115488, "BACK FOCUS POSITION"=8422304, "TRIGGER CONNECTOR"=1066432, "TRIGGER SOURCE"=1066144, "OUTPUT TRIGGER SOURCE"=1852576, "TRIGGER GLOBAL EXPOSURE"=2049680, "FIRST TRIGGER BEHAVIOR"=2049696, "CHANNEL SYNC"=1852352, "READOUT DIRECTION"=4211904, "PRE HSYNC COUNT"=1852704] ("Parameter")
                n69 = event-data() -> ("NewVal"=w373:sgl)  [unwired: 1 in, 3 out]
                n70 = call <userlib>:"tm_setparameter_a.vi"("error in (no error)"=w379, "Value in"=w373, "Parameter"=w380, "Handle in"=w378) -> ("error out"=w377:errorcluster, "Handle out"=w376:u32)  [unwired: 6 in]
                n71 = call <userlib>:"tm_getparameter_a.vi"("error in (no error)"=w377, "Parameter"=w380, "Handle in"=w376) -> ("error out"=w374:errorcluster, "Handle out"=w375:u32)  [unwired: 6 in, 1 out]
              }
              event "Trigger Mode": Value Change {
                w392 = 1 items=["Snap", "Sequence"] ("Capture mode")
                n72 = event-data() -> ("NewVal"=w386:sgl)  [unwired: 1 in, 4 out]
                n73 = call <userlib>:"tm_stopcapture.vi"("error in (no error)"=w396, "Handle in"=w397) -> ("error out"=w399:errorcluster, "Handle out"=w398:u32)  [unwired: 8 in]
                n74 = call <userlib>:"tm_unpreparecapture.vi"("error in (no error)"=w399, "Handle in"=w398) -> ("error out"=w395:errorcluster, "Handle out"=w394:u32)  [unwired: 8 in]
                n75 = call <userlib>:"tm_setpropertyvalue.vi"("error in (no error)"=w395, "Value in"=w386, "Property ID"=u32 1049104, "Handle in"=w394) -> ("error out"=w390:errorcluster, "Handle out"=w393:u32)  [unwired: 6 in]
                n76 = call <userlib>:"tm_preparecapture.vi"("Capture mode"=w392, "Handle in"=w393) -> ("Buffer Info"=w391:T7, "Handle out"=w389:u32)  [unwired: 6 in, 2 out]
                n77 = call <userlib>:"tm_startcapture_b.vi"("error in (no error)"=w390, "Handle in"=w389) -> ("error out"=w387:errorcluster, "Handle out"=w388:u32)  [unwired: 8 in]
              }
              event "Readout Direction": Value Change {
                w413 = 1 items=["Snap", "Sequence"] ("Capture mode")
                w406 = u32 4211904 items=["SENSOR MODE"=4212128, "CCD MODE"=4212384, "READOUT MODE"=4211872, "ACTIVE VIEW INDEX"=4343136, "BITS PER CHANNEL"=4342976, "IMAGE PIXEL TYPE"=4343296, "BINNING"=4215968, "EXPOSURE TIME"=2049184, "CONTRAST GAIN"=3163312, "CONTRAST OFFSET"=3163328, "LIGHT MODE"=2114720, "SENSITIVITY"=2114992, "PHOTON IMAGING MODE"=2115200, "HIGH DYNAMIC RANGE MODE"=3163360, "WHITE BALANCE"=3163568, "TEMPERATURE"=2115232, "TEMPERATURE TARGET"=2115264, "SENSOR COOLER FAN"=2115296, "LINEBUNDLE HEIGHT"=4212192, "MECHANICAL SHUTTER"=2115488, "BACK FOCUS POSITION"=8422304, "TRIGGER CONNECTOR"=1066432, "TRIGGER SOURCE"=1066144, "OUTPUT TRIGGER SOURCE"=1852576, "TRIGGER GLOBAL EXPOSURE"=2049680, "FIRST TRIGGER BEHAVIOR"=2049696, "CHANNEL SYNC"=1852352, "READOUT DIRECTION"=4211904, "PRE HSYNC COUNT"=1852704] ("Parameter")
                n78 = event-data() -> ("NewVal"=w405:sgl)  [unwired: 1 in, 3 out]
                n79 = call <userlib>:"tm_stopcapture.vi"("error in (no error)"=w418, "Handle in"=w415) -> ("error out"=w419:errorcluster, "Handle out"=w414:u32)  [unwired: 8 in]
                n80 = call <userlib>:"tm_unpreparecapture.vi"("error in (no error)"=w419, "Handle in"=w414) -> ("error out"=w417:errorcluster, "Handle out"=w416:u32)  [unwired: 8 in]
                n81 = call <userlib>:"tm_setparameter_a.vi"("error in (no error)"=w417, "Value in"=w405, "Parameter"=w406, "Handle in"=w416) -> ("error out"=w410:errorcluster, "Handle out"=w409:u32)  [unwired: 6 in]
                n82 = call <userlib>:"tm_preparecapture.vi"("error in (no error)"=w410, "Capture mode"=w413, "Handle in"=w409) -> ("error out"=w411:errorcluster, "Handle out"=w412:u32)  [unwired: 5 in, 2 out]
                n83 = call <userlib>:"tm_startcapture_b.vi"("error in (no error)"=w411, "Handle in"=w412) -> ("error out"=w407:errorcluster, "Handle out"=w408:u32)  [unwired: 8 in]
              }
              event "Camera Readout Mode", "Slit Width / Lines": Value Change {
                w430 = 1 items=["Snap", "Sequence"] ("Capture mode")
                n84 = event-data() -> ()  [unwired: 1 in, 4 out]
                n85 = call <userlib>:"tm_stopcapture.vi"("error in (no error)"=w436, "Handle in"=w437) -> ("error out"=w438:errorcluster, "Handle out"=w434:u32)  [unwired: 8 in]
                n86 = call <userlib>:"tm_unpreparecapture.vi"("error in (no error)"=w438, "Handle in"=w434) -> ("error out"=w429:errorcluster, "Handle out"=w435:u32)  [unwired: 8 in]
                n87 = call <userlib>:"tm_setpropertyvalue.vi"("error in (no error)"=w429, "Value in"="Camera Readout Mode", "Property ID"=u32 4194832, "Handle in"=w435) -> ("error out"=w439:errorcluster, "Handle out"=w440:u32)  [unwired: 6 in]
                n88 = case shown="12" "Camera Readout Mode" {
                  tunnel: w440 -> [w451 w458]
                  tunnel: [w450 w453] -> w433
                  tunnel: w439 -> [w448 w463]
                  tunnel: [w447 w463] -> w431
                  frame 1, Default {
                    n89 = local read "Exposure"() -> (w449:dbl)
                    n90 = call <userlib>:"tm_setpropertyvalue.vi"("error in (no error)"=w448, "Value in"=w449, "Property ID"=u32 2031888, "Handle in"=w451) -> ("error out"=w447:errorcluster, "Handle out"=w450:u32)  [unwired: 6 in]
                  }
                  frame 12 {
                    n91 = local read "Exposure"() -> (w462:dbl)
                    n92 = local read "SVW"() -> (w460:i32)
                    n93 = formula code="slitExpos=frameInter*LW/(LinesToReadout\n+10+LW);\nlineInter = slitExpos / LW;"("frameInter"=w462, "LW"="Slit Width / Lines", "LinesToReadout"=w460) -> ("slitExpos"=w454:dbl, "lineInter"=w457:dbl)
                    n94 = call <userlib>:"tm_setpropertyvalue.vi"("Value in"=w457, "Property ID"=u32 4208720, "Handle in"=w458) -> ("Handle out"=w456:u32)  [unwired: 7 in, 1 out]
                    n95 = call <userlib>:"tm_setpropertyvalue.vi"("Value in"=w454, "Property ID"=u32 2031888, "Handle in"=w456) -> ("Handle out"=w453:u32)  [unwired: 7 in, 1 out]
                  }
                }
                n96 = call <userlib>:"tm_preparecapture.vi"("error in (no error)"=w431, "Capture mode"=w430, "Handle in"=w433) -> ("error out"=w426:errorcluster, "Buffer Info"=w432:T7, "Handle out"=w428:u32)  [unwired: 5 in, 1 out]
                n97 = call <userlib>:"tm_startcapture_b.vi"("error in (no error)"=w426, "Handle in"=w428) -> ("error out"=w425:errorcluster, "Handle out"=w427:u32)  [unwired: 8 in]
              }
              event "Ram Record": Value Change {
                n98 = event-data() -> ()  [unwired: 1 in, 5 out]
                n99 = case shown="True" "Ram Record" {
                  tunnel: w477 -> [w481 w504]
                  tunnel: w476 -> [w480 w501]
                  tunnel: [w481 w487] -> w475
                  tunnel: [w480 w489] -> w474
                  tunnel: [w479 w488] -> w470
                  tunnel: w469 -> [w479 _]
                  tunnel: w467 -> [_ w492]
                  tunnel: [_ w490] -> w466
                  tunnel: w465 -> [_ w486]
                  tunnel: w464 -> [_ w482]
                  frame False {
                  }
                  frame True {
                    w498 = 0 items=["Snap", "Sequence"] ("Capture mode")
                    # "Max 2500"
                    n100 = Flush Queue(queue=w492) -> (queue out=w491:refnum<queue>)  [unwired: 1 in, 2 out]
                    n101 = call <userlib>:"tm_stopcapture.vi"("error in (no error)"=w504, "Handle in"=w501) -> ("error out"=w503:errorcluster, "Handle out"=w502:u32)  [unwired: 8 in]
                    n102 = call <userlib>:"tm_unpreparecapture.vi"("error in (no error)"=w503, "Handle in"=w502) -> ("error out"=w499:errorcluster, "Handle out"=w500:u32)  [unwired: 8 in]
                    n103 = call <userlib>:"tm_preparecapture.vi"("error in (no error)"=w499, "Frames"="Frames", "Capture mode"=w498, "Handle in"=w500) -> ("error out"=w497:errorcluster, "Buffer Info"=w495:T7, "Handle out"=w496:u32)  [unwired: 4 in, 1 out]
                    n104 = Bundle By Name(cluster=w482, "State"=Stack_Track."Start Sequence", "Stack Number"=0, "Image"=w486) -> (w483:T3)
                    n105 = Enqueue Element(queue=w491, element=w483) -> (queue out=w493:refnum<queue>)  [unwired: 2 in, 2 out]
                    n106 = case shown="No Error" w497 {
                      selector: w497 -> [w529 w550]
                      tunnel: w496 -> [w528 w551]
                      tunnel: "Frames" -> [w524 _]
                      tunnel: [w509 w547] -> w489
                      tunnel: w495 -> [w525 _]
                      tunnel: [w508 w549] -> w487
                      tunnel: w493 -> [w523 w545]
                      tunnel: w482 -> [w522 _]
                      tunnel: [w507 w545] -> _
                      tunnel: [FALSE ("value") w559] -> w490
                      tunnel: [w506 w548] -> w488
                      frame No Error {
                        w514 = 1 items=["Snap", "Sequence"] ("Capture mode")
                        # "Frames in RAM"
                        n107 = call <userlib>:"tm_startcapture_b.vi"("error in (no error)"=w529, "Handle in"=w528) -> ("error out"=w526:errorcluster, "Handle out"=w527:u32)  [unwired: 8 in]
                        n108 = for {
                          N: w524 -> [_]
                          tunnel: w527 -> [w544]
                          tunnel: w526 -> [w543]
                          tunnel: w525 -> [w540]
                          tunnel: [w539] -> w520
                          tunnel: [w538] -> w519
                          tunnel: w523 -> [w536]
                          tunnel: Stack_Track."Collecting" ("Enum") -> [w534]
                          tunnel: w522 -> [w532]
                          tunnel: [w531] -> w513
                          i -> [w533]
                          n109 = call <userlib>:"tm_waitnextframe.vi"("error in (no error)"=w543, "Handle in"=w544) -> ("error out"=w541:errorcluster, "Frame Index"=→"Frame Index":i32, "Handle out"=w542:u32)  [unwired: 6 in, 1 out]
                          n110 = call <userlib>:"tm_getframe_a.vi"("error in (no error)"=w541, "Frame Index"=w533, "Buffer Info"=w540, "Handle in"=w542) -> ("error out"=w538:errorcluster, "Data 16"=w530:u16[][], "Handle out"=w539:u32)  [unwired: 3 in, 2 out]
                          n111 = Bundle By Name(cluster=w532, "State"=w534, "Stack Number"=w533, "Image"=w530) -> (w535:T3)
                          n112 = Enqueue Element(queue=w536, element=w535) -> (queue out=w531:refnum<queue>)  [unwired: 2 in, 2 out]
                        }
                        n113 = call <userlib>:"tm_stopcapture.vi"("error in (no error)"=w519, "Handle in"=w520) -> ("error out"=w517:errorcluster, "Handle out"=w518:u32)  [unwired: 8 in]
                        n114 = call <userlib>:"tm_unpreparecapture.vi"("error in (no error)"=w517, "Handle in"=w518) -> ("error out"=w516:errorcluster, "Handle out"=w515:u32)  [unwired: 8 in]
                        n115 = Enqueue Element(queue=w513, element=T3 {"State"=enum."End", "Stack Number"=0, "Image"=[]} ("input cluster")) -> (queue out=w507:refnum<queue>)  [unwired: 2 in, 2 out]
                        n116 = call <userlib>:"tm_preparecapture.vi"("error in (no error)"=w516, "Capture mode"=w514, "Handle in"=w515) -> ("error out"=w511:errorcluster, "Buffer Info"=w506:T7, "Handle out"=w510:u32)  [unwired: 5 in, 1 out]
                        n117 = call <userlib>:"tm_startcapture_b.vi"("error in (no error)"=w511, "Handle in"=w510) -> ("error out"=w508:errorcluster, "Handle out"=w509:u32)  [unwired: 8 in]
                      }
                      frame Error {
                        w554 = 1 items=["Snap", "Sequence"] ("Capture mode")
                        # "Prepare camera failure, likely too many frames in stack"
                        n118 = One Button Dialog(message="Too many frames in stack", button name ("OK")="OK") -> (true=w559:bool)
                        n119 = call <userlib>:"tm_stopcapture.vi"("error in (no error)"=w550, "Handle in"=w551) -> ("error out"=w557:errorcluster, "Handle out"=w558:u32)  [unwired: 8 in]
                        n120 = call <userlib>:"tm_unpreparecapture.vi"("error in (no error)"=w557, "Handle in"=w558) -> ("error out"=w556:errorcluster, "Handle out"=w555:u32)  [unwired: 8 in]
                        n121 = Enqueue Element(queue=w545, element=T3 {"State"=enum."Idle", "Stack Number"=0, "Image"=[]} ("input cluster")) -> ()  [unwired: 2 in, 3 out]
                        n122 = call <userlib>:"tm_preparecapture.vi"("error in (no error)"=w556, "Capture mode"=w554, "Handle in"=w555) -> ("error out"=w553:errorcluster, "Buffer Info"=w548:T7, "Handle out"=w552:u32)  [unwired: 5 in, 1 out]
                        n123 = call <userlib>:"tm_startcapture_b.vi"("error in (no error)"=w553, "Handle in"=w552) -> ("error out"=w549:errorcluster, "Handle out"=w547:u32)  [unwired: 8 in]
                      }
                    }
                  }
                }
              }
              event "HardDisk Record": Value Change {
                n124 = event-data() -> ()  [unwired: 1 in, 5 out]
                n125 = case shown="True" "HardDisk Record" {
                  tunnel: w574 -> [w577 w593]
                  tunnel: w573 -> [w576 w590]
                  tunnel: [w577 w580] -> w572
                  tunnel: [w576 w582] -> w571
                  tunnel: [w575 w581] -> w567
                  tunnel: w566 -> [w575 _]
                  tunnel: w564 -> [_ w578]
                  tunnel: [_ w583] -> w563
                  frame False {
                  }
                  frame True {
                    w587 = 0 items=["Snap", "Sequence"] ("Capture mode")
                    # "Max 50"
                    n126 = call <userlib>:"tm_stopcapture.vi"("error in (no error)"=w593, "Handle in"=w590) -> ("error out"=w592:errorcluster, "Handle out"=w591:u32)  [unwired: 8 in]
                    n127 = call <userlib>:"tm_unpreparecapture.vi"("error in (no error)"=w592, "Handle in"=w591) -> ("error out"=w588:errorcluster, "Handle out"=w589:u32)  [unwired: 8 in]
                    n128 = call <userlib>:"tm_preparecapture.vi"("error in (no error)"=w588, "Frames"="Frames", "Capture mode"=w587, "Handle in"=w589) -> ("error out"=w586:errorcluster, "Buffer Info"=w584:T7, "Handle out"=w585:u32)  [unwired: 4 in, 1 out]
                    n129 = case shown="No Error" w586 {
                      selector: w586 -> [w618 w631]
                      tunnel: w585 -> [w604 w632]
                      tunnel: [w607 w628] -> w582
                      tunnel: w584 -> [w615 _]
                      tunnel: [w606 w630] -> w580
                      tunnel: [FALSE ("value") w640] -> w583
                      tunnel: [w605 w629] -> w581
                      tunnel: "Frames" -> [w601 _]
                      tunnel: w578 -> [w595 w626]
                      frame No Error {
                        w610 = 1 items=["Snap", "Sequence"] ("Capture mode")
                        n130 = call <userlib>:"tm_startrecorder.vi"("frames"=w601, "File"="Temp", "Handle in"=w604) -> ("Handle out"=w603:u32)  [unwired: 7 in, 1 out]
                        n131 = call <userlib>:"tm_startcapture_b.vi"("error in (no error)"=w618, "Handle in"=w603) -> ("error out"=w616:errorcluster, "Handle out"=w617:u32)  [unwired: 8 in]
                        n132 = while {
                          tunnel: w617 -> [w624]
                          tunnel: w616 -> [w623]
                          tunnel: w615 -> [_]
                          tunnel: [w625] -> w613
                          tunnel: w601 -> [w620]
                          stop <- w621 stop-if-true
                          n133 = Wait (ms)(milliseconds to wait=u32 50) -> ()  [unwired: 1 out]
                          n134 = call <userlib>:"tm_getrecorderstatus.vi"("error in (no error)"=w623, "Handle"=w624) -> ("error out"=w625:errorcluster, "Count"=w619:i32)  [unwired: 6 in, 2 out]
                          n135 = Equal?(x=w619, y=w620) -> (x = y?=w621:bool)
                        }
                        n136 = call <userlib>:"tm_stopcapture.vi"("error in (no error)"=w613) -> ("error out"=w600:errorcluster, "Handle out"=w599:u32)  [unwired: 9 in]
                        n137 = call <userlib>:"tm_stoprecorder.vi"("error in (no error)"=w600, "Handle in"=w599) -> ("error out"=w597:errorcluster, "Handle out"=w598:u32)  [unwired: 8 in]
                        n138 = Enqueue Element(queue=w595, element=T3 {"State"=enum."Read Disk", "Stack Number"=0, "Image"=[]}, error in (no error)=w597) -> (error out=w596:errorcluster)  [unwired: 1 in, 2 out]
                        n139 = call <userlib>:"tm_unpreparecapture.vi"("error in (no error)"=w596, "Handle in"=w598) -> ("error out"=w612:errorcluster, "Handle out"=w611:u32)  [unwired: 8 in]
                        n140 = call <userlib>:"tm_preparecapture.vi"("error in (no error)"=w612, "Capture mode"=w610, "Handle in"=w611) -> ("error out"=w609:errorcluster, "Buffer Info"=w605:T7, "Handle out"=w608:u32)  [unwired: 5 in, 1 out]
                        n141 = call <userlib>:"tm_startcapture_b.vi"("error in (no error)"=w609, "Handle in"=w608) -> ("error out"=w606:errorcluster, "Handle out"=w607:u32)  [unwired: 8 in]
                      }
                      frame Error {
                        w635 = 1 items=["Snap", "Sequence"] ("Capture mode")
                        # "Prepare camera failure, likely too many frames in stack"
                        n142 = One Button Dialog(message="Too many frames in stack", button name ("OK")="OK") -> (true=w640:bool)
                        n143 = call <userlib>:"tm_stopcapture.vi"("error in (no error)"=w631, "Handle in"=w632) -> ("error out"=w638:errorcluster, "Handle out"=w639:u32)  [unwired: 8 in]
                        n144 = call <userlib>:"tm_unpreparecapture.vi"("error in (no error)"=w638, "Handle in"=w639) -> ("error out"=w637:errorcluster, "Handle out"=w636:u32)  [unwired: 8 in]
                        n145 = Enqueue Element(queue=w626, element=T3 {"State"=enum."STOP", "Stack Number"=0, "Image"=[]} ("input cluster")) -> ()  [unwired: 2 in, 3 out]
                        n146 = call <userlib>:"tm_preparecapture.vi"("error in (no error)"=w637, "Capture mode"=w635, "Handle in"=w636) -> ("error out"=w634:errorcluster, "Buffer Info"=w629:T7, "Handle out"=w633:u32)  [unwired: 5 in, 1 out]
                        n147 = call <userlib>:"tm_startcapture_b.vi"("error in (no error)"=w634, "Handle in"=w633) -> ("error out"=w630:errorcluster, "Handle out"=w628:u32)  [unwired: 8 in]
                      }
                    }
                  }
                }
              }
              event "Scan Mode": Value Change {
                w643 = u32 4211872 items=["SENSOR MODE"=4212128, "CCD MODE"=4212384, "READOUT MODE"=4211872, "ACTIVE VIEW INDEX"=4343136, "BITS PER CHANNEL"=4342976, "IMAGE PIXEL TYPE"=4343296, "BINNING"=4215968, "EXPOSURE TIME"=2049184, "CONTRAST GAIN"=3163312, "CONTRAST OFFSET"=3163328, "LIGHT MODE"=2114720, "SENSITIVITY"=2114992, "PHOTON IMAGING MODE"=2115200, "HIGH DYNAMIC RANGE MODE"=3163360, "WHITE BALANCE"=3163568, "TEMPERATURE"=2115232, "TEMPERATURE TARGET"=2115264, "SENSOR COOLER FAN"=2115296, "LINEBUNDLE HEIGHT"=4212192, "MECHANICAL SHUTTER"=2115488, "BACK FOCUS POSITION"=8422304, "TRIGGER CONNECTOR"=1066432, "TRIGGER SOURCE"=1066144, "OUTPUT TRIGGER SOURCE"=1852576, "TRIGGER GLOBAL EXPOSURE"=2049680, "FIRST TRIGGER BEHAVIOR"=2049696, "CHANNEL SYNC"=1852352, "READOUT DIRECTION"=4211904, "PRE HSYNC COUNT"=1852704] ("Parameter")
                w658 = 1 items=["Snap", "Sequence"] ("Capture mode")
                n148 = event-data() -> ("NewVal"=w648:dbl)  [unwired: 1 in, 2 out]
                n149 = call <userlib>:"tm_stopcapture.vi"("error in (no error)"=w659, "Handle in"=w660) -> ("error out"=w661:errorcluster, "Handle out"=w662:u32)  [unwired: 8 in]
                n150 = call <userlib>:"tm_unpreparecapture.vi"("error in (no error)"=w661, "Handle in"=w662) -> ("error out"=w646:errorcluster, "Handle out"=w647:u32)  [unwired: 8 in]
                n151 = call <userlib>:"tm_setparameter_a.vi"("error in (no error)"=w646, "Value in"=w648, "Parameter"=w643, "Handle in"=w647) -> ("error out"=w645:errorcluster, "Handle out"=w644:u32)  [unwired: 6 in]
                n152 = call <userlib>:"tm_getparameter_a.vi"("error in (no error)"=w645, "Parameter"=w643, "Handle in"=w644) -> ("error out"=w651:errorcluster, "Value out"=w650:dbl, "Handle out"=w649:u32)  [unwired: 6 in]
                n153 = local write "SMD"(w650) -> ()
                n154 = call <userlib>:"tm_preparecapture.vi"("error in (no error)"=w651, "Capture mode"=w658, "Handle in"=w649) -> ("error out"=w656:errorcluster, "Buffer Info"=w653:T7, "Handle out"=w657:u32)  [unwired: 5 in, 1 out]
                n155 = call <userlib>:"tm_startcapture_b.vi"("error in (no error)"=w656, "Handle in"=w657) -> ("error out"=w655:errorcluster, "Handle out"=w654:u32)  [unwired: 8 in]
              }
              event "Binning": Value Change {
                w667 = u32 4215968 items=["BINNING"=4215968, "BITS PER CHANNEL"=2, "ACTIVE VIEW INDEX"=3, "CCD MODE"=4, "SENSOR MODE"=5, "READOUT MODE"=6, "EXPOSURE TIME"=7, "CONTRAST GAIN"=8, "CONTRAST OFFSET"=9, "LIGHT MODE"=10, "SENSITIVITY"=11, "WHITE BALANCE"=12, "PHOTON IMAGING MODE"=13, "HIGH DYNAMIC RANGE MODE"=14, "TRIGGER SOURCE"=15, "TRIGGER ACTIVE"=16, "TRIGGER MODE"=17, "TRIGGER POLARITY"=18, "TRIGGER GLOBAL EXPOSURE"=19, "FIRST TRIGGER BEHAVIOR"=20, "TRIGGER TIMES"=21, "OUTPUT TRIGGER POLARITY"=22, "OUTPUT TRIGGER DELAY"=23, "OUTPUT TRIGGER PERIOD"=24, "TEMPERATURE"=25, "TEMPERATURE TARGET"=26, "SENSOR COOLER FAN"=27, "MECHANICAL SHUTTER"=28, "BACK FOCUS POSITION"=29, "FRAMEBUNDLE MODE"=30, "FRAMEBUNDLE NUMBER"=31, "LINEBUNDLE HEIGHT"=32, "TRIGGER CONNECTOR"=33, "IMAGE PIXEL TYPE"=34, "OUTPUT TRIGGER KIND"=35, "READOUT DIRECTION"=36, "CHANNEL SYNC"=37] ("Parameter")
                w706 = 1 items=["Snap", "Sequence"] ("Capture mode")
                n156 = event-data() -> ("NewVal"=w668:u16)  [unwired: 1 in, 2 out]
                n157 = call <userlib>:"tm_stopcapture.vi"("error in (no error)"=w675, "Handle in"=w676) -> ("error out"=w673:errorcluster, "Handle out"=w674:u32)  [unwired: 8 in]
                n158 = call <userlib>:"tm_unpreparecapture.vi"("error in (no error)"=w673, "Handle in"=w674) -> ("error out"=w669:errorcluster, "Handle out"=w666:u32)  [unwired: 8 in]
                n159 = call <userlib>:"tm_setparameter_a.vi"("error in (no error)"=w669, "Value in"=w668, "Parameter"=w667, "Handle in"=w666) -> ("error out"=w670:errorcluster, "Handle out"=w671:u32)  [unwired: 6 in]
                n160 = call <userlib>:"tm_getarea_a.vi"("error in (no error)"=w670, "Handle in"=w671) -> ("error out"=w694:errorcluster, "V Offset"=w696:T6, "H Offset"=w695:T6, "Handle out"=w693:u32, "H Width"=w697:T6, "V Width"=w698:T6)  [unwired: 4 in]
                n161 = Unbundle By Name(w695) -> ("Value"=w689:i32, "Minimum"=w692:i32, "Maximum"=w691:i32, "Increment"=w690:i32)
                n162 = Unbundle By Name(w696) -> ("Value"=w679:i32, "Minimum"=w688:i32, "Maximum"=w687:i32, "Increment"=w686:i32)
                n163 = Unbundle By Name(w697) -> ("Value"=w678:i32, "Minimum"=w685:i32, "Maximum"=w684:i32, "Increment"=w683:i32)
                n164 = Unbundle By Name(w698) -> ("Value"=w677:i32, "Minimum"=w682:i32, "Maximum"=w681:i32, "Increment"=w680:i32)
                n165 = property on="H Offset" class="DigNum (strict)"("Value"=w689, "Minimum"=w692, "Maximum"=w691, "Increment"=w690) -> ()  [unwired: 2 in, 2 out]
                n166 = property on="V Offset" class="DigNum (strict)"("Value"=w679, "Minimum"=w688, "Maximum"=w687, "Increment"=w686) -> ()  [unwired: 2 in, 2 out]
                n167 = property on="H Width" class="DigNum (strict)"("Value"=w678, "Minimum"=w685, "Maximum"=w684, "Increment"=w683) -> ()  [unwired: 2 in, 2 out]
                n168 = property on="V Width" class="DigNum (strict)"("Value"=w677, "Minimum"=w682, "Maximum"=w681, "Increment"=w680) -> ()  [unwired: 2 in, 2 out]
                n169 = local write "SHO"(w689) -> ()
                n170 = local write "SVO"(w679) -> ()
                n171 = local write "SHW"(w678) -> ()
                n172 = local write "SVW"(w677) -> ()
                n173 = call <userlib>:"tm_preparecapture.vi"("error in (no error)"=w694, "Capture mode"=w706, "Handle in"=w693) -> ("error out"=w704:errorcluster, "Buffer Info"=w701:T7, "Handle out"=w705:u32)  [unwired: 5 in, 1 out]
                n174 = call <userlib>:"tm_startcapture_b.vi"("error in (no error)"=w704, "Handle in"=w705) -> ("error out"=w703:errorcluster, "Handle out"=w702:u32)  [unwired: 8 in]
              }
              event "H Offset", "H Width", "V Offset", "V Width": Value Change {
                w751 = 1 items=["Snap", "Sequence"] ("Capture mode")
                n175 = event-data() -> ()  [unwired: 1 in, 4 out]
                n176 = call <userlib>:"tm_stopcapture.vi"("error in (no error)"=w713, "Handle in"=w714) -> ("error out"=w711:errorcluster, "Handle out"=w712:u32)  [unwired: 8 in]
                n177 = local read "H Offset"() -> (w717:i32)
                n178 = local read "H Width"() -> (w718:i32)
                n179 = local read "V Offset"() -> (w719:i32)
                n180 = local read "V Width"() -> (w716:i32)
                n181 = call <userlib>:"tm_unpreparecapture.vi"("error in (no error)"=w711, "Handle in"=w712) -> ("error out"=w709:errorcluster, "Handle out"=w710:u32)  [unwired: 8 in]
                n182 = Bundle("H Offset"=w717, "V Offset"=w719, "H Width"=w718, "V Width"=w716) -> (w715:T8)  [unwired: 1 in]
                n183 = call <userlib>:"tm_setarea.vi"("error in (no error)"=w709, "Sub Region"=w715, "Handle in"=w710) -> ("error out"=w720:errorcluster, "Handle out"=w721:u32)  [unwired: 7 in]
                n184 = call <userlib>:"tm_getarea_a.vi"("error in (no error)"=w720, "Handle in"=w721) -> ("error out"=w739:errorcluster, "V Offset"=w741:T6, "H Offset"=w740:T6, "Handle out"=w738:u32, "H Width"=w742:T6, "V Width"=w743:T6)  [unwired: 4 in]
                n185 = Unbundle By Name(w740) -> ("Value"=w734:i32, "Minimum"=w737:i32, "Maximum"=w736:i32, "Increment"=w735:i32)
                n186 = Unbundle By Name(w741) -> ("Value"=w724:i32, "Minimum"=w733:i32, "Maximum"=w732:i32, "Increment"=w731:i32)
                n187 = Unbundle By Name(w742) -> ("Value"=w723:i32, "Minimum"=w730:i32, "Maximum"=w729:i32, "Increment"=w728:i32)
                n188 = Unbundle By Name(w743) -> ("Value"=w722:i32, "Minimum"=w727:i32, "Maximum"=w726:i32, "Increment"=w725:i32)
                n189 = property on="H Offset" class="DigNum (strict)"("Value"=w734, "Minimum"=w737, "Maximum"=w736, "Increment"=w735) -> ()  [unwired: 2 in, 2 out]
                n190 = property on="V Offset" class="DigNum (strict)"("Value"=w724, "Minimum"=w733, "Maximum"=w732, "Increment"=w731) -> ()  [unwired: 2 in, 2 out]
                n191 = property on="H Width" class="DigNum (strict)"("Value"=w723, "Minimum"=w730, "Maximum"=w729, "Increment"=w728) -> ()  [unwired: 2 in, 2 out]
                n192 = property on="V Width" class="DigNum (strict)"("Value"=w722, "Minimum"=w727, "Maximum"=w726, "Increment"=w725) -> ()  [unwired: 2 in, 2 out]
                n193 = local write "SHO"(w734) -> ()
                n194 = local write "SVO"(w724) -> ()
                n195 = local write "SHW"(w723) -> ()
                n196 = local write "SVW"(w722) -> ()
                n197 = call <userlib>:"tm_preparecapture.vi"("error in (no error)"=w739, "Capture mode"=w751, "Handle in"=w738) -> ("error out"=w749:errorcluster, "Buffer Info"=w746:T7, "Handle out"=w750:u32)  [unwired: 5 in, 1 out]
                n198 = call <userlib>:"tm_startcapture_b.vi"("error in (no error)"=w749, "Handle in"=w750) -> ("error out"=w748:errorcluster, "Handle out"=w747:u32)  [unwired: 8 in]
              }
            }
            n199 = local read "stop"() -> (w255:bool)
            n200 = Unbundle By Name(w264) -> ("status"=w277:bool)
            n201 = Compound Arithmetic op=OR(w277, w255, w259) -> (w276:bool)
          }
        }
        frame Enabled {
        }
      }
      n202 = while {
        tunnel: w9 -> [w104]
        tunnel: w10 -> [w107]
        tunnel: w15 -> [w103]
        shift-right: [w102] -> _
        shift-left: w14 -> [w105]
        shift-right: [w101] -> w8
        shift-left: w13 -> [w106]
        tunnel: w12 -> [w100]
        tunnel: [w99] -> w7
        stop <- w94 stop-if-true
        n203 = Dequeue Element(queue=w107, timeout in ms (-1)=1) -> (element=w95:T2, timed out?=w97:bool)  [unwired: 1 in, 2 out]
        n204 = case shown="True" w97 {
          tunnel: [w108 CameraControlTypeDef."Idle" ("Enum")] -> w96
          tunnel: w95 -> [w108 _]
          frame False {
          }
          frame True {
          }
        }
        n205 = case shown="\"Idle\", Default" w96 {
          selector: w96 -> [_ _ w188 _ _]
          tunnel: w106 -> [w112 w113 _ w226 w243]
          tunnel: w105 -> [w111 w115 _ w211 w235]
          tunnel: w104 -> [_ _ _ _ w241]
          tunnel: w103 -> [_ _ _ _ w240]
          tunnel: [w111 w115 w126 w211 w235] -> w102
          tunnel: [w112 w113 w116 w212 w234] -> w101
          tunnel: w100 -> [w110 w114 w185 w225 w231]
          tunnel: [w110 w114 w125 w210 w233] -> w99
          frame "Ram Record" {
          }
          frame "HardDisk Record" {
          }
          frame "Disengage Update" {
            w129 = 1 items=["Snap", "Sequence"] ("Capture mode")
            w132 = u32 4215968 items=["BINNING"=4215968, "BITS PER CHANNEL"=2, "ACTIVE VIEW INDEX"=3, "CCD MODE"=4, "SENSOR MODE"=5, "READOUT MODE"=6, "EXPOSURE TIME"=7, "CONTRAST GAIN"=8, "CONTRAST OFFSET"=9, "LIGHT MODE"=10, "SENSITIVITY"=11, "WHITE BALANCE"=12, "PHOTON IMAGING MODE"=13, "HIGH DYNAMIC RANGE MODE"=14, "TRIGGER SOURCE"=15, "TRIGGER ACTIVE"=16, "TRIGGER MODE"=17, "TRIGGER POLARITY"=18, "TRIGGER GLOBAL EXPOSURE"=19, "FIRST TRIGGER BEHAVIOR"=20, "TRIGGER TIMES"=21, "OUTPUT TRIGGER POLARITY"=22, "OUTPUT TRIGGER DELAY"=23, "OUTPUT TRIGGER PERIOD"=24, "TEMPERATURE"=25, "TEMPERATURE TARGET"=26, "SENSOR COOLER FAN"=27, "MECHANICAL SHUTTER"=28, "BACK FOCUS POSITION"=29, "FRAMEBUNDLE MODE"=30, "FRAMEBUNDLE NUMBER"=31, "LINEBUNDLE HEIGHT"=32, "TRIGGER CONNECTOR"=33, "IMAGE PIXEL TYPE"=34, "OUTPUT TRIGGER KIND"=35, "READOUT DIRECTION"=36, "CHANNEL SYNC"=37] ("Parameter")
            w159 = u32 4211872 items=["SENSOR MODE"=4212128, "CCD MODE"=4212384, "READOUT MODE"=4211872, "ACTIVE VIEW INDEX"=4343136, "BITS PER CHANNEL"=4342976, "IMAGE PIXEL TYPE"=4343296, "BINNING"=4215968, "EXPOSURE TIME"=2049184, "CONTRAST GAIN"=3163312, "CONTRAST OFFSET"=3163328, "LIGHT MODE"=2114720, "SENSITIVITY"=2114992, "PHOTON IMAGING MODE"=2115200, "HIGH DYNAMIC RANGE MODE"=3163360, "WHITE BALANCE"=3163568, "TEMPERATURE"=2115232, "TEMPERATURE TARGET"=2115264, "SENSOR COOLER FAN"=2115296, "LINEBUNDLE HEIGHT"=4212192, "MECHANICAL SHUTTER"=2115488, "BACK FOCUS POSITION"=8422304, "TRIGGER CONNECTOR"=1066432, "TRIGGER SOURCE"=1066144, "OUTPUT TRIGGER SOURCE"=1852576, "TRIGGER GLOBAL EXPOSURE"=2049680, "FIRST TRIGGER BEHAVIOR"=2049696, "CHANNEL SYNC"=1852352, "READOUT DIRECTION"=4211904, "PRE HSYNC COUNT"=1852704] ("Parameter")
            w172 = u32 4211904 items=["SENSOR MODE"=4212128, "CCD MODE"=4212384, "READOUT MODE"=4211872, "ACTIVE VIEW INDEX"=4343136, "BITS PER CHANNEL"=4342976, "IMAGE PIXEL TYPE"=4343296, "BINNING"=4215968, "EXPOSURE TIME"=2049184, "CONTRAST GAIN"=3163312, "CONTRAST OFFSET"=3163328, "LIGHT MODE"=2114720, "SENSITIVITY"=2114992, "PHOTON IMAGING MODE"=2115200, "HIGH DYNAMIC RANGE MODE"=3163360, "WHITE BALANCE"=3163568, "TEMPERATURE"=2115232, "TEMPERATURE TARGET"=2115264, "SENSOR COOLER FAN"=2115296, "LINEBUNDLE HEIGHT"=4212192, "MECHANICAL SHUTTER"=2115488, "BACK FOCUS POSITION"=8422304, "TRIGGER CONNECTOR"=1066432, "TRIGGER SOURCE"=1066144, "OUTPUT TRIGGER SOURCE"=1852576, "TRIGGER GLOBAL EXPOSURE"=2049680, "FIRST TRIGGER BEHAVIOR"=2049696, "CHANNEL SYNC"=1852352, "READOUT DIRECTION"=4211904, "PRE HSYNC COUNT"=1852704] ("Parameter")
            w183 = u32 1049104 ("Property ID")
            n206 = call <userlib>:"tm_stopcapture.vi"("error in (no error)"=w185, "Handle in"=w188) -> ("error out"=w186:errorcluster, "Handle out"=w187:u32)  [unwired: 8 in]
            n207 = call <userlib>:"tm_unpreparecapture.vi"("error in (no error)"=w186, "Handle in"=w187) -> ("error out"=w174:errorcluster, "Handle out"=w182:u32)  [unwired: 8 in]
            n208 = local read "Trigger Mode"() -> (w184:sgl)
            n209 = call <userlib>:"tm_setpropertyvalue.vi"("error in (no error)"=w174, "Value in"=w184, "Property ID"=w183, "Handle in"=w182) -> ("error out"=w175:errorcluster)  [unwired: 6 in, 1 out]
            n210 = local read "Readout Direction"() -> (w179:sgl)
            n211 = call <userlib>:"tm_getpropertyvalue.vi"("error in (no error)"=w175, "Property ID"=w183, "Handle in"=w182) -> ("error out"=w176:errorcluster, "Value in"=w181:sgl, "Handle out"=w180:u32)  [unwired: 6 in]
            n212 = call <userlib>:"tm_setparameter_a.vi"("error in (no error)"=w176, "Value in"=w179, "Parameter"=w172, "Handle in"=w180) -> ("error out"=w177:errorcluster, "Handle out"=w178:u32)  [unwired: 6 in]
            n213 = local write "Trigger Mode"(w181) -> ()
            n214 = local read "Camera Readout Mode"() -> (w168:u16)
            n215 = call <userlib>:"tm_getparameter_a.vi"("error in (no error)"=w177, "Parameter"=w172, "Handle in"=w178) -> ("error out"=w170:errorcluster, "Value out"=w173:dbl, "Handle out"=w171:u32)  [unwired: 6 in]
            n216 = local write "Readout Direction"(w173) -> ()
            n217 = call <userlib>:"tm_setpropertyvalue.vi"("error in (no error)"=w170, "Value in"=w168, "Property ID"=u32 4194832, "Handle in"=w171) -> ("error out"=w166:errorcluster, "Handle out"=w167:u32)  [unwired: 6 in]
            n218 = case shown="12" w168 {
              tunnel: [w192 w196] -> w165
              tunnel: w167 -> [w191 w197]
              tunnel: w166 -> [w190 w196]
              tunnel: [w189 w195] -> w163
              frame 1, Default {
                n219 = local read "Exposure"() -> (w193:dbl)
                n220 = call <userlib>:"tm_setpropertyvalue.vi"("error in (no error)"=w190, "Value in"=w193, "Property ID"=u32 2031888, "Handle in"=w191) -> ("error out"=w192:errorcluster, "Handle out"=w189:u32)  [unwired: 6 in]
              }
              frame 12 {
                n221 = local read "Exposure"() -> (w205:dbl)
                n222 = local read "SVW"() -> (w203:i32)
                n223 = formula code="slitExpos=frameInter*LW/(LinesToReadout\n+10+LW);\nlineInter = slitExpos / LW;"("frameInter"=w205, "LW"="Slit Width / Lines 2", "LinesToReadout"=w203) -> ("slitExpos"=w198:dbl, "lineInter"=w201:dbl)
                n224 = call <userlib>:"tm_setpropertyvalue.vi"("Value in"=w201, "Property ID"=u32 4208720, "Handle in"=w197) -> ("Handle out"=w200:u32)  [unwired: 7 in, 1 out]
                n225 = call <userlib>:"tm_setpropertyvalue.vi"("Value in"=w198, "Property ID"=u32 2031888, "Handle in"=w200) -> ("Handle out"=w195:u32)  [unwired: 7 in, 1 out]
              }
            }
            n226 = local read "Scan Mode"() -> (w162:dbl)
            n227 = call <userlib>:"tm_setparameter_a.vi"("error in (no error)"=w165, "Value in"=w162, "Parameter"=w159, "Handle in"=w163) -> ("error out"=w164:errorcluster, "Handle out"=w160:u32)  [unwired: 6 in]
            n228 = call <userlib>:"tm_getparameter_a.vi"("error in (no error)"=w164, "Parameter"=w159, "Handle in"=w160) -> ("error out"=w158:errorcluster, "Value out"=w161:dbl, "Handle out"=w157:u32)  [unwired: 6 in]
            n229 = local write "Scan Mode"(w161) -> ()
            n230 = local read "Binning"() -> (w156:u16)
            n231 = call <userlib>:"tm_setparameter_a.vi"("error in (no error)"=w158, "Value in"=w156, "Parameter"=w132, "Handle in"=w157) -> ("error out"=w135:errorcluster, "Handle out"=w134:u32)  [unwired: 6 in]
            n232 = call <userlib>:"tm_getparameter_a.vi"("error in (no error)"=w135, "Parameter"=w132, "Handle in"=w134) -> ("error out"=w131:errorcluster, "Value out"=w133:dbl, "Handle out"=w119:u32)  [unwired: 6 in]
            n233 = local write "Binning"(w133) -> ()
            n234 = local read "V Width"() -> (w121:i32)
            n235 = local read "V Offset"() -> (w123:i32)
            n236 = local read "H Width"() -> (w122:i32)
            n237 = local read "H Offset"() -> (w124:i32)
            n238 = Bundle("H Offset"=w124, "V Offset"=w123, "H Width"=w122, "V Width"=w121) -> (w120:T8)  [unwired: 1 in]
            n239 = call <userlib>:"tm_setarea.vi"("Sub Region"=w120, "Handle in"=w119) -> ("Handle out"=w118:u32)  [unwired: 8 in, 1 out]
            n240 = call <userlib>:"tm_getarea_a.vi"("error in (no error)"=w131, "Handle in"=w118) -> ("error out"=w130:errorcluster, "V Offset"=w138:T6, "H Offset"=w139:T6, "Handle out"=w117:u32, "H Width"=w137:T6, "V Width"=w136:T6)  [unwired: 4 in]
            n241 = Unbundle By Name(w139) -> ("Value"=w143:i32, "Minimum"=w140:i32, "Maximum"=w141:i32, "Increment"=w142:i32)
            n242 = Unbundle By Name(w138) -> ("Value"=w153:i32, "Minimum"=w144:i32, "Maximum"=w145:i32, "Increment"=w146:i32)
            n243 = Unbundle By Name(w137) -> ("Value"=w154:i32, "Minimum"=w147:i32, "Maximum"=w148:i32, "Increment"=w149:i32)
            n244 = Unbundle By Name(w136) -> ("Value"=w155:i32, "Minimum"=w150:i32, "Maximum"=w151:i32, "Increment"=w152:i32)
            n245 = property on="H Offset" class="DigNum (strict)"("Value"=w143, "Minimum"=w140, "Maximum"=w141, "Increment"=w142) -> ()  [unwired: 2 in, 2 out]
            n246 = property on="V Offset" class="DigNum (strict)"("Value"=w153, "Minimum"=w144, "Maximum"=w145, "Increment"=w146) -> ()  [unwired: 2 in, 2 out]
            n247 = property on="H Width" class="DigNum (strict)"("Value"=w154, "Minimum"=w147, "Maximum"=w148, "Increment"=w149) -> ()  [unwired: 2 in, 2 out]
            n248 = property on="V Width" class="DigNum (strict)"("Value"=w155, "Minimum"=w150, "Maximum"=w151, "Increment"=w152) -> ()  [unwired: 2 in, 2 out]
            n249 = local write "SHO"(w143) -> ()
            n250 = local write "SVO"(w153) -> ()
            n251 = local write "SHW"(w154) -> ()
            n252 = local write "SVW"(w155) -> ()
            n253 = call <userlib>:"tm_preparecapture.vi"("error in (no error)"=w130, "Capture mode"=w129, "Handle in"=w117) -> ("error out"=w128:errorcluster, "Buffer Info"=w126:T7, "Handle out"=w127:u32)  [unwired: 5 in, 1 out]
            n254 = call <userlib>:"tm_startcapture_b.vi"("error in (no error)"=w128, "Handle in"=w127) -> ("error out"=w125:errorcluster, "Handle out"=w116:u32)  [unwired: 8 in]
          }
          frame "Update" {
            w216 = u32 1066144 items=["SENSOR MODE"=4212128, "CCD MODE"=4212384, "READOUT MODE"=4211872, "ACTIVE VIEW INDEX"=4343136, "BITS PER CHANNEL"=4342976, "IMAGE PIXEL TYPE"=4343296, "BINNING"=4215968, "EXPOSURE TIME"=2049184, "CONTRAST GAIN"=3163312, "CONTRAST OFFSET"=3163328, "LIGHT MODE"=2114720, "SENSITIVITY"=2114992, "PHOTON IMAGING MODE"=2115200, "HIGH DYNAMIC RANGE MODE"=3163360, "WHITE BALANCE"=3163568, "TEMPERATURE"=2115232, "TEMPERATURE TARGET"=2115264, "SENSOR COOLER FAN"=2115296, "LINEBUNDLE HEIGHT"=4212192, "MECHANICAL SHUTTER"=2115488, "BACK FOCUS POSITION"=8422304, "TRIGGER CONNECTOR"=1066432, "TRIGGER SOURCE"=1066144, "OUTPUT TRIGGER SOURCE"=1852576, "TRIGGER GLOBAL EXPOSURE"=2049680, "FIRST TRIGGER BEHAVIOR"=2049696, "CHANNEL SYNC"=1852352, "READOUT DIRECTION"=4211904, "PRE HSYNC COUNT"=1852704] ("Parameter")
            w221 = u32 4191424 items=["SENSOR MODE"=4212128, "CCD MODE"=4212384, "READOUT MODE"=4211872, "ACTIVE VIEW INDEX"=4343136, "BITS PER CHANNEL"=4342976, "IMAGE PIXEL TYPE"=4343296, "BINNING"=4215968, "EXPOSURE TIME"=2049184, "CONTRAST GAIN"=3163312, "CONTRAST OFFSET"=3163328, "LIGHT MODE"=2114720, "SENSITIVITY"=2114992, "PHOTON IMAGING MODE"=2115200, "HIGH DYNAMIC RANGE MODE"=3163360, "WHITE BALANCE"=3163568, "TEMPERATURE"=2115232, "TEMPERATURE TARGET"=2115264, "SENSOR COOLER FAN"=2115296, "LINEBUNDLE HEIGHT"=4212192, "MECHANICAL SHUTTER"=2115488, "BACK FOCUS POSITION"=8422304, "TRIGGER CONNECTOR"=1066432, "TRIGGER SOURCE"=1066144, "OUTPUT TRIGGER SOURCE"=1852576, "TRIGGER GLOBAL EXPOSURE"=2049680, "FIRST TRIGGER BEHAVIOR"=2049696, "CHANNEL SYNC"=1852352, "READOUT DIRECTION"=4211904, "PRE HSYNC COUNT"=1852704, "INTERNAL LINE SPEED"=4191408, "INTERNAL LINE INVERVAL"=4191424] ("Parameter")
            w222 = u32 2049184 items=["SENSOR MODE"=4212128, "CCD MODE"=4212384, "READOUT MODE"=4211872, "ACTIVE VIEW INDEX"=4343136, "BITS PER CHANNEL"=4342976, "IMAGE PIXEL TYPE"=4343296, "BINNING"=4215968, "EXPOSURE TIME"=2049184, "CONTRAST GAIN"=3163312, "CONTRAST OFFSET"=3163328, "LIGHT MODE"=2114720, "SENSITIVITY"=2114992, "PHOTON IMAGING MODE"=2115200, "HIGH DYNAMIC RANGE MODE"=3163360, "WHITE BALANCE"=3163568, "TEMPERATURE"=2115232, "TEMPERATURE TARGET"=2115264, "SENSOR COOLER FAN"=2115296, "LINEBUNDLE HEIGHT"=4212192, "MECHANICAL SHUTTER"=2115488, "BACK FOCUS POSITION"=8422304, "TRIGGER CONNECTOR"=1066432, "TRIGGER SOURCE"=1066144, "OUTPUT TRIGGER SOURCE"=1852576, "TRIGGER GLOBAL EXPOSURE"=2049680, "FIRST TRIGGER BEHAVIOR"=2049696, "CHANNEL SYNC"=1852352, "READOUT DIRECTION"=4211904, "PRE HSYNC COUNT"=1852704] ("Parameter")
            n255 = local read "EXP"() -> (w227:dbl)
            n256 = call <userlib>:"tm_setparameter_a.vi"("error in (no error)"=w225, "Value in"=w227, "Parameter"=w222, "Handle in"=w226) -> ("error out"=w229:errorcluster, "Handle out"=w223:u32)  [unwired: 6 in]
            n257 = call <userlib>:"tm_getparameter_a.vi"("error in (no error)"=w229, "Parameter"=w222, "Handle in"=w223) -> ("error out"=w206:errorcluster, "Value out"=w228:dbl, "Handle out"=w224:u32)  [unwired: 6 in]
            n258 = local read "Internal Line Interval"() -> (w214:dbl)
            n259 = local write "EXP"(w228) -> ()
            n260 = call <userlib>:"tm_setparameter_a.vi"("error in (no error)"=w206, "Value in"=w214, "Parameter"=w221, "Handle in"=w224) -> ("error out"=w207:errorcluster, "Handle out"=w220:u32)  [unwired: 6 in]
            n261 = call <userlib>:"tm_getparameter_a.vi"("error in (no error)"=w207, "Parameter"=w221, "Handle in"=w220) -> ("error out"=w208:errorcluster, "Value out"=w219:dbl, "Handle out"=w218:u32)  [unwired: 6 in]
            n262 = local write "Internal Line Interval"(w219) -> ()
            n263 = local read "Trigger Source"() -> (w213:sgl)
            n264 = call <userlib>:"tm_setparameter_a.vi"("error in (no error)"=w208, "Value in"=w213, "Parameter"=w216, "Handle in"=w218) -> ("error out"=w209:errorcluster, "Handle out"=w217:u32)  [unwired: 6 in]
            n265 = call <userlib>:"tm_getparameter_a.vi"("error in (no error)"=w209, "Parameter"=w216, "Handle in"=w217) -> ("error out"=w210:errorcluster, "Value out"=w215:dbl, "Handle out"=w212:u32)  [unwired: 6 in]
            n266 = local write "Trigger Source"(w215) -> ()
          }
          frame "Idle", Default {
            n267 = call <userlib>:"tm_waitnextframe.vi"("error in (no error)"=w231, "Timeout"=100, "Handle in"=w243) -> ("error out"=w230:errorcluster, "Handle out"=w242:u32)  [unwired: 5 in, 2 out]
            n268 = call <userlib>:"tm_getframe_a.vi"("error in (no error)"=w230, "Buffer Info"=w235, "Handle in"=w242) -> ("error out"=w233:errorcluster, "Data 16"=w237:u16[][], "Handle out"=w234:u32)  [unwired: 4 in, 2 out]
            n269 = Bundle By Name(cluster=w240, "State"=Stack_Track."Idle", "Stack Number"=0, "Image"=w237) -> (w236:T3)
            n270 = Enqueue Element(queue=w241, element=w236) -> ()  [unwired: 2 in, 3 out]
          }
        }
        n271 = local read "stop"() -> (w94:bool)
      }
      n272 = while {
        tunnel: w9 -> [w767]
        shift-right: [w763] -> _
        shift-left: _ -> [w761]
        shift-right: [w759] -> _
        shift-left: _ -> [w760]
        shift-right: [w757] -> _
        shift-left: _ -> [w753]
        stop <- w762 stop-if-true
        n273 = Dequeue Element(queue=w767) -> (element=w766:T3, timed out?=w754:bool)  [unwired: 2 in, 2 out]
        n274 = Unbundle By Name(w766) -> ("State"=w765:T1, "Stack Number"=w764:i32, "Image"=w755:u16[][])
        "State" <- w765
        n275 = case shown="False" w754 {
          tunnel: w755 -> [w769 w771]
          tunnel: [w769 w770] -> w756
          tunnel: [w768 w771] -> w757
          tunnel: w753 -> [w768 w770]
          frame False {
          }
          frame True {
          }
        }
        "Image" <- w756
        n276 = case shown="\"Idle\"" w765 {
          tunnel: w764 -> [_ _ _ _ _ _]
          tunnel: [w774 w791 _ _ _ _] -> w763
          tunnel: w761 -> [_ w792 w798 _ _ _]
          tunnel: [FALSE _ _ _ TRUE _] -> w762
          tunnel: w756 -> [w772 w793 _ _ _ _]
          tunnel: w760 -> [_ w790 w796 w808 w833 w835]
          tunnel: [w775 w789 w797 w804 w833 w835] -> w759
          tunnel: "Path" -> [w778 _ _ w810 _ _]
          frame "Start Sequence" {
            # "Public tiff library"
            # "Get path and open file"
            n277 = Equal?(x=w778, y=path "") -> (x = y?=w780:bool)
            n278 = case shown="True" w780 {
              tunnel: w778 -> [w782 _]
              tunnel: [w782 w785] -> w777
              frame False {
              }
              frame True {
                n279 = call "File Dialog"("pattern (all files)"=".tiff", "pattern label"="Tiff Image") -> ("selected path"=w785:path)  [unwired: 10 in, 3 out]
              }
            }
            n280 = case shown="False" "AutoIncrement" {
              tunnel: w777 -> [w786 w788]
              tunnel: [w786 w787] -> w773
              frame False {
              }
              frame True {
                n281 = call "4Digit File Incrementer.vi"("path"=w788) -> ("appended path"=w787:path)  [unwired: 10 in]
              }
            }
            n282 = call-poly "CTIFFNewFileAndStyle.vi"("image"=w772, "output_file"=w773) -> ("error"=w775:errorcluster, "CTIFF"=w774:i64)  [unwired: 8 in]
            n283 = local write "Path"(w773) -> ()
          }
          frame "Collecting" {
            # "Add Image to write scan line"
            n284 = call-poly "CTIFFAddNewPage.vi"("error"=w790, "image"=w793, "CTIFF"=w792) -> ("error"=w789:errorcluster, "CTIFF"=w791:i64)  [unwired: 7 in]
            n285 = property on="Ram Record" class="Bool (strict)"("DisabledEnum"=T4."Disabled and Grayed Out" ("Disabled"), "BoolText.Text"="Saving" ("Boolean Text.Text")) -> ()  [unwired: 2 in, 2 out]
          }
          frame "End" {
            (unwired) FALSE
            # "Close image file, reset capturing button"
            n286 = call "CTIFFWriteAndClose.vi"("error"=w796, "CTIFF"=w798) -> ("error"=w797:errorcluster)  [unwired: 9 in]
            n287 = property on="Ram Record" class="Bool (strict)"("BoolText.Text"="OK" ("Boolean Text.Text"), "DisabledEnum"=T4."Enabled" ("Disabled")) -> ()  [unwired: 2 in, 2 out]
          }
          frame "Read Disk" {
            n288 = local read "Temp"() -> (w805:path)
            n289 = call <userlib>:"tm_opendcimgfile.vi"("Path"=w805) -> ("Total Frames"=w811:i32, "File Handle"=w812:u32)  [unwired: 8 in, 1 out]
            n290 = for {
              N: w811 -> [_]
              tunnel: w810 -> [w820]
              shift-right: [w818] -> w806
              shift-left: i64 0 ("CTIFF") -> [w819]
              tunnel: [w817] -> w807
              tunnel: w808 -> [w816]
              shift-right: [w822] -> w801
              shift-left: w812 -> [w823]
              i -> [w814]
              n291 = Equal To 0?(x=w814) -> (x = 0?=w821:bool)
              n292 = call <userlib>:"tm_getdcimgframe.vi"("error in (no error)"=w816, "Frame Index"=w814, "File Handle in"=w823) -> ("error out"=w815:errorcluster, "Data"=w813:u16[][], "File Handle out"=w822:u32)  [unwired: 5 in, 1 out]
              n293 = local write "Image"(w813) -> ()
              n294 = case shown="True" w821 {
                tunnel: w820 -> [_ w832]
                tunnel: w813 -> [w824 w831]
                tunnel: w819 -> [w828 _]
                tunnel: [w827 w830] -> w818
                tunnel: [w826 w829] -> w817
                tunnel: w815 -> [w825 _]
                frame False {
                  n295 = call-poly "CTIFFAddNewPage.vi"("error"=w825, "image"=w824, "CTIFF"=w828) -> ("error"=w826:errorcluster, "CTIFF"=w827:i64)  [unwired: 7 in]
                }
                frame True {
                  n296 = call-poly "CTIFFNewFileAndStyle.vi"("image"=w831, "output_file"=w832) -> ("error"=w829:errorcluster, "CTIFF"=w830:i64)  [unwired: 8 in]
                }
              }
              "Frame Index" <- w814
            }
            n297 = call "CTIFFWriteAndClose.vi"("error"=w807, "CTIFF"=w806) -> ("error"=w803:errorcluster)  [unwired: 9 in]
            n298 = call <userlib>:"tm_closedcimgfile.vi"("error in (no error)"=w803, "File Handle"=w801) -> ("error out"=w802:errorcluster)  [unwired: 9 in]
            n299 = Delete(path (use dialog)=w805, error in=w802) -> (error out=w804:errorcluster)  [unwired: 3 in, 2 out]
          }
          frame "STOP" {
          }
          frame "Idle" {
          }
        }
      }
      n300 = while {
        tunnel: w10 -> [w91]
        stop <- "stop" stop-if-true
        n301 = event shown="[0] Timeout" {
          selector: _ -> [_]
          dyn-events: _ -> [_]
          timeout: _ -> [_]
          tunnel: w91 -> [w93]
          event Timeout {
            n302 = event-data() -> ()  [unwired: 1 in, 3 out]
            n303 = Enqueue Element(queue=w93, element=CameraControlTypeDef."Idle") -> ()  [unwired: 2 in, 3 out]
          }
        }
      }
      n304 = call <userlib>:"tm_stopcapture.vi"("error in (no error)"=w7, "Handle in"=w8) -> ("error out"=w59:errorcluster, "Handle out"=w60:u32)  [unwired: 8 in]
      n305 = call <userlib>:"tm_unpreparecapture.vi"("error in (no error)"=w59, "Handle in"=w60) -> ("error out"=w58:errorcluster, "Handle out"=w61:u32)  [unwired: 8 in]
      n306 = call <userlib>:"tm_closecamera.vi"("error in (no error)"=w58, "Handle in"=w61) -> ("error out"=w87:errorcluster)  [unwired: 9 in]
      n307 = call <userlib>:"tm_deinitialize.vi"("error in (no error)"=w87) -> ("error out"=w86:errorcluster)  [unwired: 10 in]
    }
  }
  "error out" <- w3
